vi "H2O_DIAL_NCAR_4CH_v4.07.vi"() -> ()   [LabVIEW 2012]
uses:
  C:/Users/H2ODial/Desktop/Shared Telescope WV DIAL Code/Libraries and VIs/PowerMeterCommands.dll
  Libraries and VIs/PowerMeterCommands.dll
  <vilib>/DAQmx/write.llb/DAQmx Write (Digital 1D Bool NChan 1Samp 1Line).vi
  <vilib>/DAQmx/miscellaneous.llb/DAQmx Fill In Error Info.vi
  <vilib>/Analysis/baseanly.llb/Mean (DBL).vi
  AMCS_Data.vi
  Libraries and VIs/Scalar_Data.vi
  <vilib>/Analysis/NI_AALBase.lvlib
  Libraries and VIs/Scalar_Data_2.vi
  Libraries and VIs/Scalar_Data_4.vi
  Libraries and VIs/Scalar_Data_3.vi
  Libraries and VIs/CLDevIFace.dll
panel:
  in  "Cancel Offline":bool
  out "AMCS_Profile":i32=9505
  out "FileHour":i32=21
  out "L_Count":i32=24
  out "sigma_off_total":dbl[](array[numeric])=[5.235525125067343e-25, 5.206358319245337e-25, 5.177318750524933e-25, 5.148406424862825e-25, 5.119621341127451e-25, 5.090963491196627e-25, 5.062432860011865e-25, 5.034029425635027e-25, 5.005753159352157e-25, 4.977604025706667e-25, 4.949581982592347e-25, 4.921686981325722e-25, 4.893918966711095e-25, 4.866277877122191e-25, 4.8387636445644285e-25, 4.811376194764721e-25, 4.784115447230487e-25, 4.756981315339233e-25, 4.729973706394386e-25, 4.703092521721628e-25, 4.6763376567211625e-25, 4.6497090009594435e-25, 4.623206438225019e-25, 4.596829846622293e-25, 4.57057909862005e-25, 4.544454061150213e-25, 4.518454595652437e-25, 4.492580558158126e-25, 4.4668317993693425e-25, 4.441208164702635e-25, 4.41570949437918e-25, 4.390335623482575e-25, 4.365086382028137e-25, 4.339961595028071e-25, 4.314961082547237e-25, 4.290084659777996e-25, 4.2653321370993085e-25, 4.240703320135042e-25, 4.216198009811418e-25, 4.191816002426457e-25, 4.16755708969195e-25, 4.143421058805604e-25, 4.1194076924960845e-25, 4.095516769084665e-25, 4.0717480625238245e-25, 4.0481013424706545e-25, 4.0245763743206737e-25, 4.001172919260011e-25, 3.977890734322512e-25, 3.9547295724256756e-25, 3.931689182419048e-25, 3.908769309139365e-25, 3.8859696934393876e-25, 3.863290072236815e-25, 3.840730178557474e-25, 3.8182897415734565e-25, 3.7959684866403156e-25, 3.773766135338825e-25, 3.7516824055099053e-25, 3.729717011286995e-25, 3.707869663137923e-25, 3.686140067893342e-25, 3.664527928779591e-25, 3.643032945453827e-25, 3.621654814033011e-25, 3.600393227122229e-25, 3.579247873843723e-25, 3.5582184398664743e-25, 3.5373046074361216e-25, 3.5165060553938904e-25, 3.4958224592064764e-25, 3.475253490990589e-25, 3.454798819536632e-25, 3.4344581103303625e-25, 3.414231025576395e-25, 3.394117224218377e-25, 3.37411636196096e-25, 3.3542280912885406e-25, 3.3344520614845767e-25, 3.3147879186525413e-25, 3.295235305730259e-25, 3.275793862509532e-25, 3.2564632256504646e-25, 3.237243028702917e-25, 3.2181329021119735e-25, 3.1991324732434905e-25, 3.180241366390581e-25, 3.161459202790299e-25, 3.142785600633377e-25, 3.1242201750825597e-25, 3.1057625382770893e-25, 3.0874122993477767e-25, 3.0691690644282785e-25, 3.051032436660927e-25, 3.0330020162078266e-25, 3.0150774002602592e-25, 2.997258183045521e-25, 2.979543955833093e-25, 2.961934306943937e-25, 2.944428821752431e-25, 2.9270270826932477e-25, 2.909728669267514e-25, 2.8925331580414936e-25, 2.875440122654977e-25, 2.8584491338173137e-25, 2.841559759313169e-25, 2.8247715639976386e-25, 2.80808410980223e-25, 2.791496955724979e-25, 2.775009657833479e-25, 2.7586217692567447e-25, 2.742332840183121e-25, 2.7261424178518227e-25, 2.710050046547509e-25, 2.6940552675881075e-25, 2.6781576193155516e-25, 2.6623566370876434e-25, 2.646651853260364e-25, 2.6310427971768174e-25, 2.615528995144771e-25, 2.600109970428841e-25, 2.5847852432207883e-25, 2.569554330624564e-25, 2.554416746633416e-25, 2.5393720020962457e-25, 2.5244196047033826e-25, 2.5095590589459477e-25, 2.4947898660936654e-25, 2.480111524155541e-25, 2.4655235278440513e-25, 2.451025368544176e-25, 2.436616534266772e-25, 2.422296509605852e-25, 2.408064775697375e-25, 2.3939208101763006e-25, 2.3798640871112015e-25, 2.365894076971971e-25, 2.352010246556833e-25, 2.3382120589521406e-25, 2.324498973455175e-25, 2.3108704455300754e-25, 2.2973259267270024e-25, 2.283864864626908e-25, 2.270486702764721e-25, 2.257190880557015e-25, 2.2439768332388837e-25, 2.2308439917739663e-25, 2.2177917827749597e-25, 2.20481962844103e-25, 2.19192694645104e-25, 2.179113149897461e-25, 2.166377647190967e-25, 2.153719841983278e-25, 2.1411391330535246e-25, 2.1286349142540036e-25, 2.1162065743868337e-25, 2.103853497130775e-25, 2.091575060946101e-25, 2.079370638983031e-25, 2.0672395989815037e-25, 2.0551813031976677e-25, 2.0431951082869756e-25, 2.0312803652523447e-25, 2.019436419319984e-25, 2.0076626098781596e-25, 1.9959582703908636e-25, 1.9843227283026113e-25, 1.9727553050009988e-25, 1.9612553156963306e-25, 1.9498220693936616e-25, 1.9384548688025462e-25, 1.9271530103114487e-25, 1.915915783921294e-25, 1.9047424731896738e-25, 1.8936323552292957e-25, 1.8825847006561212e-25, 1.8715987735714719e-25, 1.8606738315918164e-25, 1.8498091257941087e-25, 1.8390039007904753e-25, 1.8282573946936752e-25, 1.8175688392200846e-25, 1.80693745969556e-25, 1.7963624751388698e-25, 1.7858430983630522e-25, 1.7753785360393623e-25, 1.7649679888396773e-25, 1.7546106515613228e-25, 1.7443057132789558e-25, 1.7340523575155863e-25, 1.723849762422857e-25, 1.7136971010131167e-25, 1.7035935413825008e-25, 1.6935382469544605e-25, 1.6835303767796407e-25, 1.6735690858143057e-25, 1.6636535252563445e-25, 1.653782842907513e-25, 1.643956183497921e-25, 1.6341726891478545e-25, 1.624431499756322e-25, 1.6147317534796005e-25, 1.6050725871551994e-25, 1.5954531368896971e-25, 1.585872538492723e-25, 1.576329928151117e-25, 1.566824442883223e-25, 1.5573552212546758e-25, 1.5479214039898043e-25, 1.5385221346219397e-25, 1.5291565602013113e-25, 1.519823831962039e-25, 1.5105231061650234e-25, 1.5012535447460145e-25, 1.49201431624485e-25, 1.482804596459418e-25, 1.4736235693849326e-25, 1.46447042805166e-25, 1.455344375360034e-25, 1.4462446250285657e-25, 1.4371704024629248e-25, 1.4281209456557682e-25, 1.4190955061389853e-25, 1.410093350012645e-25, 1.4011137586880333e-25, 1.3921560301221658e-25, 1.3832194795253431e-25, 1.3743034404767374e-25, 1.3654072658699072e-25, 1.3565303288298996e-25, 1.3476720236918642e-25, 1.3388317669734332e-25, 1.3300089982893968e-25, 1.3212031812258562e-25, 1.3124138043688156e-25, 1.3036403820696332e-25, 1.2948824553577423e-25, 1.2861395928315612e-25, 1.2774113913410786e-25, 1.2686974768684636e-25, 1.2599975053009544e-25, 1.2513111630057894e-25, 1.2426381676023619e-25, 1.2339782685325752e-25, 1.2253312476934588e-25, 1.2166969199403071e-25, 1.2080751335374065e-25, 1.1994657705541538e-25, 1.1908687474046665e-25, 1.182284014933639e-25, 1.1737115587808914e-25, 1.1651513996305814e-25, 1.1566035931942852e-25, 1.1480682304187532e-25, 1.1395454373665928e-25, 1.1310353751750977e-25, 1.1225382399779688e-25, 1.1140542626706877e-25, 1.1055837085176348e-25, 1.097126877076807e-25, 1.0886841014622313e-25, 1.0802557481625692e-25, 1.07184221622742e-25, 1.0634439369229237e-25, 1.0550613727868173e-25, 1.0466950171251473e-25, 1.038345393031225e-25, 1.0300130526116006e-25, 1.0216985760646603e-25, 1.0134025706453978e-25, 1.0051256696943142e-25, 9.968685315566847e-26, 9.886318383691271e-26, 9.804162950309608e-26, 9.722226278487634e-26, 9.640515833439737e-26, 9.559039270504641e-26]
  out "sigma_on_total":dbl[](array[numeric])=[2.0626424870063408e-23, 2.0548386991725913e-23, 2.0469620043661083e-23, 2.039014007926666e-23, 2.0309963185763554e-23, 2.022910547933105e-23, 2.0147583096531975e-23, 2.0065412185834914e-23, 1.9982608903424648e-23, 1.9899189402652408e-23, 1.9815169828925073e-23, 1.973056631280819e-23, 1.9645394962489817e-23, 1.9559671857889236e-23, 1.9473413042995686e-23, 1.9386634520995392e-23, 1.9299352246499e-23, 1.92115821209391e-23, 1.9123339984701628e-23, 1.9034641613560593e-23, 1.894550271072393e-23, 1.8855938903179933e-23, 1.8765965734424238e-23, 1.8675598661476663e-23, 1.858485304716652e-23, 1.8493744158198464e-23, 1.8402287157379186e-23, 1.831049710049574e-23, 1.8218388932961533e-23, 1.8125977482532266e-23, 1.8033277457757753e-23, 1.794030344287124e-23, 1.78470698943209e-23, 1.7753591137085564e-23, 1.765988136004934e-23, 1.756595461410152e-23, 1.7471824808549346e-23, 1.737750570768982e-23, 1.728301092753991e-23, 1.718835393452682e-23, 1.7093548040708237e-23, 1.6998606403479167e-23, 1.690354202181418e-23, 1.6808367735172782e-23, 1.671309621933486e-23, 1.6617739987721353e-23, 1.652231138715337e-23, 1.6426822596607076e-23, 1.6331285627143943e-23, 1.623571231880846e-23, 1.614011433977554e-23, 1.6044503186999793e-23, 1.594889018281904e-23, 1.5853286475164595e-23, 1.5757703037183567e-23, 1.56621506662899e-23, 1.5566639983337563e-23, 1.5471181432924705e-23, 1.5375785282782344e-23, 1.5280461622943503e-23, 1.5185220367027678e-23, 1.5090071251272868e-23, 1.4995023834679822e-23, 1.490008749990639e-23, 1.480527145325558e-23, 1.4710584724761487e-23, 1.461603616869313e-23, 1.4521634464462555e-23, 1.4427388117922844e-23, 1.4333305460496324e-23, 1.4239394650957737e-23, 1.4145663676315014e-23, 1.4052120352758215e-23, 1.3958772326362732e-23, 1.386562707448506e-23, 1.377269190659265e-23, 1.3679973965774194e-23, 1.3587480229685293e-23, 1.349521751185974e-23, 1.340319246367332e-23, 1.331141157483609e-23, 1.3219881175450048e-23, 1.312860743690352e-23, 1.303759637488782e-23, 1.2946853848301087e-23, 1.2856385563810112e-23, 1.276619707542367e-23, 1.2676293787044932e-23, 1.2586680953306706e-23, 1.2497363683020601e-23, 1.2408346938918898e-23, 1.231963554057768e-23, 1.2231234166482255e-23, 1.2143147354716326e-23, 1.205537950536109e-23, 1.1967934882614928e-23, 1.18808176163727e-23, 1.179403170382724e-23, 1.1707581012163646e-23, 1.1621469279366376e-23, 1.1535700116662612e-23, 1.1450277010949764e-23, 1.1365203325379191e-23, 1.1280482302846387e-23, 1.119611706633001e-23, 1.1112110622106432e-23, 1.1028465860371398e-23, 1.0945185558937296e-23, 1.0862272383097774e-23, 1.0779728889052267e-23, 1.0697557524793115e-23, 1.061576063274372e-23, 1.0534340451140567e-23, 1.0453299116394038e-23, 1.0372638664219593e-23, 1.0292361031742144e-23, 1.0212468060051632e-23, 1.0132961495072904e-23, 1.0053842990094956e-23, 9.975114106406274e-24, 9.896776316950593e-24, 9.818831006241923e-24, 9.741279473284931e-24, 9.664122933306695e-24, 9.587362518136572e-24, 9.510999279944331e-24, 9.4350341911426e-24, 9.35946814739855e-24, 9.284301968408356e-24, 9.209536399550346e-24, 9.135172114369533e-24, 9.061209715316372e-24, 8.987649735342966e-24, 8.914492639894921e-24, 8.841738828863562e-24, 8.769388636455937e-24, 8.697442334770948e-24, 8.625900133437759e-24, 8.554762182711667e-24, 8.484028573306861e-24, 8.413699339425238e-24, 8.343774458768281e-24, 8.274253854911725e-24, 8.20513739808004e-24, 8.136424906498288e-24, 8.068116148476333e-24, 8.000210842753849e-24, 7.93270865979759e-24, 7.865609224179398e-24, 7.798912114328467e-24, 7.732616864864992e-24, 7.666722967246401e-24, 7.601229871485918e-24, 7.536136986062991e-24, 7.47144368084401e-24, 7.407149286604625e-24, 7.343253097014758e-24, 7.279754369538433e-24, 7.216652326491339e-24, 7.153946155744344e-24, 7.091635012419465e-24, 7.029718018888616e-24, 6.968194267085294e-24, 6.907062818145217e-24, 6.846322704177098e-24, 6.785972929020363e-24, 6.726012468678494e-24, 6.666440273317614e-24, 6.607255266717305e-24, 6.5484563482276464e-24, 6.490042392830114e-24, 6.4320122527255365e-24, 6.374364757672102e-24, 6.317098715478381e-24, 6.260212913519775e-24, 6.203706118893361e-24, 6.147577079162962e-24, 6.091824523799792e-24, 6.036447163734017e-24, 5.981443693189575e-24, 5.9268127892254286e-24, 5.872553113518711e-24, 5.818663312168178e-24, 5.765142016606135e-24, 5.711987844480541e-24, 5.659199399714517e-24, 5.60677527349843e-24, 5.554714044726636e-24, 5.503014280556554e-24, 5.451674536954151e-24, 5.400693359100156e-24, 5.3500692821650106e-24, 5.29980083168557e-24, 5.249886523936265e-24, 5.200324866659172e-24, 5.151114359286823e-24, 5.102253493524346e-24, 5.053740753912813e-24, 5.0055746177903024e-24, 4.9577535563097775e-24, 4.9102760344956494e-24, 4.8631405118766655e-24, 4.816345442421003e-24, 4.769889275599373e-24, 4.7237704559666584e-24, 4.677987424414909e-24, 4.6325386175288775e-24, 4.587422468700435e-24, 4.542637408235811e-24, 4.498181863571078e-24, 4.454054259692367e-24, 4.410253019129813e-24, 4.366776562876656e-24, 4.323623309953703e-24, 4.2807916785034235e-24, 4.238280085149713e-24, 4.196086945869007e-24, 4.15421067614052e-24, 4.112649690999126e-24, 4.0714024055659475e-24, 4.030467235085202e-24, 3.989842595058185e-24, 3.949526901559562e-24, 3.9095185718135265e-24, 3.8698160234810635e-24, 3.830417676044675e-24, 3.7913219499109044e-24, 3.752527267230076e-24, 3.7140320519806624e-24, 3.675834729967747e-24, 3.6379337290799074e-24, 3.600327479534733e-24, 3.563014413948001e-24, 3.525992967320637e-24, 3.489261577597712e-24, 3.4528186853946936e-24, 3.416662734299426e-24, 3.380792171158687e-24, 3.345205445806531e-24, 3.309901011503899e-24, 3.2748773251256216e-24, 3.240132846887192e-24, 3.205666040760562e-24, 3.171475374424784e-24, 3.1375593195130495e-24, 3.103916351630131e-24, 3.070544950370658e-24, 3.0374435993380817e-24, 3.004610786651537e-24, 2.9720450044576056e-24, 2.939744749292133e-24, 2.907708522285371e-24, 2.875934828888819e-24, 2.8444221792793013e-24, 2.813169088151738e-24, 2.7821740748481583e-24, 2.751435663542785e-24, 2.7209523832266658e-24, 2.6907227675070794e-24, 2.6607453552206828e-24, 2.631018689789545e-24, 2.601541319883231e-24, 2.5723117989072515e-24, 2.5433286855837636e-24, 2.514590543447409e-24, 2.4860959413513324e-24, 2.4578434531440932e-24, 2.4298316578731105e-24, 2.402059139807656e-24, 2.3745244883501128e-24, 2.3472262981695396e-24, 2.3201631692184444e-24, 2.2933337065889e-24, 2.2667365207963308e-24, 2.240370227526033e-24, 2.2142334477539052e-24, 2.188324807908419e-24]
  out "background start":u32=269
  in  "Tab Control 2":enum32{"WV ND far", "WV ND near"}(tab)
  out "Water Vapor Number Density":dbl[][](graph)=[[1.0639074632249623, 0.7950854451951521, 0.6871802900906222, 0.6578628096137078, 0.7135791866585837, 0.791964119748022, 0.7860957670990096, 0.7853422876996722, 0.8071252522931472, 0.8864535505893456, 1.0159198981230433, 0.9651627659284989, 0.8682042083486436, 0.9042154310622283, 0.8685330628018557, 0.7776092079248705, 0.772778664796884, 0.7959779985601635, 0.8008645625247376, 0.7172845453518656, 0.6359963863515634, 0.7577960001972899, 0.7813956634686308, 0.6712364496556374, 0.799991558752808, 0.8995446623945136, 0.8463956496056573, 0.9017639404246155, 0.6968132420137522, 0.4583190307261309, 0.9013318132552974, 0.9419840408259437, 0.2861834314217356, 0.4216587338337765, 0.874217351771625, 0.8730810394400317, 1.1849849949997056, 0.877588935205842, -0.09895312689728929, 0.2099354782570955, 0.33582425948864986, 0.3612751226151659, 0.28889957151168794, 0.27667685078031906, -0.08105679033755347, -0.25446230513135015, -0.2766196124323003, -0.18163086301089895, 0.12220991421169942, 0.48573696212417655, 0.648089394728748, 0.7347271367978115, 0.548882739398166, 0.33491079910936744, 0.6580156316208491, 0.8064375648282445, 0.8640275078789249, 0.8753236062578905, 0.6701265812361802, 0.3904351761194603, 0.24849863279105913, 0.09000958662382388, 0.265877091881824, 0.5782261463654136, 0.6582345385490979, 0.5377226976111342, 0.521998023122092, 0.49899994069903986, 0.442086244580199, 0.7757271869672275, 1.6438430791775833, 1.7725263534215783, -4.366638673239888, -6.139974535528756, -7.260343261365436, -3.647297503921928, 2.5607177071489544, -3.1758534783949344, -4.1712374154778065, -4.871973805244922, -7.278334464601457, -6.425192249591581, -2.0047084004412903, 2.3698571856595816, 7.6963844059742055, 2.29139948545028, -6.73627824143711, -2.991965195732426, 3.0525104440963333, 3.2900333489586076, -1.1469438869155248, -2.480793373210193, 2.985721257146301, 6.404469953330058, 2.223833509425413, -3.3828689101014184, -0.7090064353515616, 1.7614922219798188, -10.376535524618875, -5.53316518310933, -1.3807982250792938, -4.60098490166722, 7.202468070896515, 26.808797183465867, -5.359274301526265, 5.1064602266204036, 8.904280843443795, 5.443742898428987, 12.764870740289377, 5.608742098911494, 9.23856034631878, 13.494920524668304, -1.6256568257766502, -27.752190916852243, 4.922130515696406, 1.2918095411038983, -2.2167544171775706, 3.8512090071660414, 0.8411143725920815, 2.3628258559477175, -0.0338690724559584, 0.5037405048509485, 0.857274736311794, 0.5609093472806994, 0.38332080391643575, 1.2134171316753553, 5.4760246071133345, 10.097061664150369, 14.664568150924406, -9.066581270887879, 3.8358908500396702, -4.8511138822779785, -2.9839925207514213, 10.022780631409056, 1.4845952961432987, 1.3621427534838009, -11.797751493789379, -19.62876466384785, -15.407318505260495, 12.982964456880289, -28.114070918045577, -10.314928052994132, -14.6863478886457, -7.4678357637899575, 8.005743163091363, -4.049991074487799, 3.834478174499156, 1.9703319457006785, -18.69907677622087, -21.61726008053773, 17.044786369322896, 13.067986458307882, 5.562083807824563, -33.1062622690423, -18.99604811314825, -14.780095581334582, -9.038972930950822, 25.682641251556422, 29.060493890117453, 30.197267081841407, 0.1585102430855488, -19.120769948554525, -50.066668611302525, 6.80906230633824, -36.08725775608675, -13.983058385627226, -11.304401633639582, -45.42704769175601, 4.201427809981585, -29.24086259807242, 18.154194101391802, 22.333042820598845, 45.23184778962592, 8.205432492461684, 36.41380298442893, 31.12103406953646, 8.501419515989362, 4.038593181058191, -39.965946639630644, 23.376757826064956, -12.263734474568551, -9.673975161682188, -1.2694403063797983, 31.516249824703433, 26.931341924650482, -12.240477775714073, -9.145842740233656, 4.271762269200702, 28.58651015280052, 22.54270081951647, -10.57215914472278, -0.9151487571192986, 1.767320075481733, -8.699514625176734, -36.202725126831716, 7.3259828957797914, 20.584536573322936, 4.297763618632405, -7.114175066775342, -41.052676712996984, 4.575962205650572, -16.179022663355003, -4.304361509159662, -22.29272241704299, 5.168440976430942, -4.301060404937512, 5.910531683494024, 13.869916287008905, 3.299425512420319, -10.2596400971753, -15.98556021271673, -21.119499530599604, 10.121801879771763, 17.07162378753489, 21.60248052204745, -44.7136046984398, -69.32086239761064, -8.665106806341068, 10.787462206990869, 30.84192690886579, -62.81604147152294, 68.55391085081732, 8.457719191474123, -28.577047707128873, 38.603673426774556, 61.94525626705892, 33.58700658348496, -1.9078968009888306, -32.30145114234005, -18.09981763911342, 88.5341483784121, -53.75429796396262, -12.113128819524603, -20.864631528502642, -53.546127210198485, 19.394365608128517, 26.53767479667509, -6.401595356851402, -61.36866888555028, -67.51786171355864, 2.78000703125268, 76.33614125496274, -35.64199728183781, 4.150760130500163, -4.696052234502958, -64.62075727916867, -9.689952747671516, 30.355740029469093, 158.13941477463777, 84.62554961101615, 37.37518451892517, -19.315848810070918, 22.407516333304084, 38.17938221937312, 19.600756478441497, 45.386701820912904, 51.438745402980494, 8.749021339340636, -91.86439146049418, 9.144403904105646, -34.267323390646695, -74.3567957578877, 39.32846577092227, 50.75034914631157, -10.066496831755677, 85.8002054961762, -10.499894043979156, 14.390636790059602, 68.28171532154174, 22.15122916807249, 14.907521727984179, 71.39835561945517, 9.422251399802613, -23.7765608484535, 23.347606952235623, -72.28850134204748, 0.0, 0.0, 0.0, 0.0]]
  out "Water Vapor Number Density 2":dbl[][](graph)=[[nan, nan, nan, nan, nan, nan, nan, nan, nan, nan, nan, nan, nan, nan, nan, nan, nan, nan, nan, nan, nan, nan, nan, nan, nan, nan, nan, nan, nan, nan, nan, nan, nan, nan, nan, nan, nan, nan, nan, nan, nan, nan, nan, nan, nan, nan, nan, nan, nan, nan, nan, nan, nan, nan, nan, nan, nan, nan, nan, nan, nan, nan, nan, nan, nan, nan, nan, nan, nan, nan, nan, nan, nan, nan, nan, nan, nan, nan, nan, nan, nan, nan, nan, nan, nan, nan, nan, nan, nan, nan, nan, nan, nan, nan, nan, nan, nan, nan, nan, nan, nan, nan, nan, nan, nan, nan, nan, nan, nan, nan, nan, nan, nan, nan, nan, nan, nan, nan, nan, nan, nan, nan, nan, nan, nan, nan, nan, nan, nan, nan, nan, nan, nan, nan, nan, nan, nan, nan, nan, nan, nan, nan, nan, nan, nan, nan, nan, nan, nan, nan, nan, nan, nan, nan, nan, nan, nan, nan, nan, nan, nan, nan, nan, nan, nan, nan, nan, nan, nan, nan, nan, nan, nan, nan, nan, nan, nan, nan, nan, nan, nan, nan, nan, nan, nan, nan, nan, nan, nan, nan, nan, nan, nan, nan, nan, nan, nan, nan, nan, nan, nan, nan, nan, nan, nan, nan, nan, nan, nan, nan, nan, nan, nan, nan, nan, nan, nan, nan, nan, nan, nan, nan, nan, nan, nan, nan, nan, nan, nan, nan, nan, nan, nan, nan, nan, nan, nan, nan, nan, nan, nan, nan, nan, nan, nan, nan, nan, nan, nan, nan, nan, nan, nan, nan, nan, nan, nan, nan, nan, nan, nan, nan, nan, nan, nan, nan, nan, nan, nan, nan, nan, nan, nan, nan, nan, nan, 0.0, 0.0, 0.0, 0.0]] caption="Water Vapor Number Density"
  out "RingBuffer offline near":dbl[][](array[numeric])
  out "RingBuffer aerosol near":dbl[][](array[numeric])
  in  "?":T1(tab)=enum."Raw Counts far"
  out "NRB":dbl[][](graph)=[[0.00021949387338662354, 0.0012644243666972022, 0.003588214032197759, 0.007224875605591026, 0.01195486448906066, 0.017431459045268816, 0.02324525277374715, 0.028802949441434758, 0.03357339059910846, 0.03782380503740098, 0.04151485605543974, 0.04515843930280387, 0.049063338651475254, 0.05265022207418093, 0.05575153288521212, 0.058504265927874735, 0.06054542510466426, 0.06174893486130328, 0.06273751305790501, 0.0632643954466035, 0.06351151944448351, 0.06357989044996755, 0.06341560380273549, 0.06303851009419217, 0.062470398076431455, 0.06280916033724494, 0.06322756790340872, 0.06364161839774003, 0.06419606813751108, 0.06488643226694854, 0.06547481871569719, 0.06547690406532276, 0.0653459113875375, 0.06474035391034692, 0.06486724045628954, 0.06495721309884349, 0.06533471884747548, 0.06616972815999793, 0.06638610910810476, 0.06655916600871534, 0.06537078233011287, 0.06602313200264284, 0.07317302762243715, 0.09749970595442206, 0.16406250986720886, 0.2791180302249938, 0.4176438777801052, 0.6802666334717046, 1.1591238150403569, 1.8560464374847874, 3.875101405163791, 6.174829462839288, 7.153508037509122, 6.549121280175305, 4.477651124476559, 2.2218355272416597, 0.7640138940197323, 0.38355427091296046, 0.22127538753969628, 0.15301899733856175, 0.11710012281226226, 0.08146079585564299, 0.055184033492043434, 0.037862430693885785, 0.034092862578169306, 0.05242220252049839, 0.07432678147202534, 0.07994648052250543, 0.07740338358404796, 0.09601527433306305, 0.13781740302265783, 0.16817436004198102, 0.17204903952050793, 0.14666788769173048, 0.08534420683870735, 0.026147036283789102, 0.004856085115782482, 0.0011524972448401112, -0.0013581678605637906, -0.0003334964710556502, -0.00010807353538194676, -0.003124612121326412, -0.004336002492278915, -0.0014014221205421228, 0.0027475954822278555, 0.003000058320868829, -0.000784026500043395, -0.0036292638303861017, -0.0018994070353000377, -0.0022502258539117076, -0.0033235236994120262, -0.0002667745861222975, 0.002857604546389024, 0.0024085602442003792, 0.0008948278806142738, -0.004348316485827131, -0.0036123162720960353, -0.001093692801835954, -7.606460251392899e-05, 0.0001995662750162021, -0.0032458877310182544, -0.0067049146072067555, -0.011255959074133778, -0.0075100285269975465, -1.5715830895250584e-05, 0.0014521797234306707, 0.0017698492925668126, -0.0021134242858882064, -0.006198461561210931, 0.002272948224295056, 0.01583894655602962, 0.03911679247954582, 0.05065155756276627, 0.03434974415408211, 0.016131693983398827, 0.0015259742615324821, -0.0029356412127107072, 0.006441985833132487, 0.0067535033006338955, -0.002232846099778923, 0.0030169480576232905, 0.006072797187070327, 0.00840132753763888, 0.025648255839425066, 0.07154886818880388, 0.13144237654754948, 0.14147442902347296, 0.10060890346164576, 0.06881876829844959, 0.04548498306360664, 0.018363981113472608, 0.007178133641252553, 0.0006471905285573144, 0.00013082291360446007, -0.0003868015765336126, -0.0008319776309399116, -0.0032372953366313776, 0.003079661264735281, 0.0007528035169903232, -0.006857440598945683, -0.011190829128121376, -0.020132237433723756, -0.012449768687672693, -0.004430467301130137, -0.0045588153304884195, -0.007187731694288056, -0.008552841137992364, -0.0057034422030721, -0.0038995755277612646, 0.0026406996122382968, 0.0019898633505103873, -0.012364667965739512, -0.004352753118895328, -0.0026819703918430173, -0.005247351813261463, 0.008252545743437438, -0.00042554135370181706, -0.013261247816825816, -0.01437057771837057, -0.017613037229624345, -0.015329648358374798, -0.013109901231006636, -0.024991290073243147, -0.01028335129982454, -0.005170113537865864, -0.011255810708455646, -0.004015231795578576, -0.005471582128283474, 0.0004116530263236128, 0.002979866875647862, 0.0142463354607509, 0.015327191442677624, 0.005148032069807082, 0.008324711549857047, -0.0007954919041935178, -0.0104941333208857, -0.0038654329070212587, -0.0065438045583597225, -0.0146355737553841, -0.005870623016356129, -0.010346492671299242, -0.01279570499844253, 0.002657403663372611, -0.003185200259090592, -0.002189979195384867, 0.0029918256232875457, -0.0005483203986729846, 0.0005374071696337536, -0.018466354202582292, -0.03392773745655944, -0.020303701319439753, -0.014882696897406955, -0.006601732618584244, -0.007475045766542423, -0.013725356228314145, -0.0030666031317952477, 0.007536028196976982, -0.0018876410045178442, -0.013447494563607994, 0.008337497509276084, -0.0013373777621936394, -0.029592197421304763, -0.01056697775939752, 0.0018521820948973538, 0.0037341208592153487, 0.0007124540469122575, -0.012785942256115651, -0.00506390285966855, 0.005057410403679166, -0.020597837150005866, -0.041524722796550874, -0.005153764699711019, 0.012402834478974131, -0.010763999846621129, -0.019650264880285036, -0.009746865677268082, -0.013379913325527208, -0.02005193275862931, -0.017425758044107502, -0.01839015378175284, -0.014960704010900442, -0.002568131262422916, -0.01101894224132209, -0.017396108976988567, 0.01716737049069364, 0.026947396830469546, 0.002415797307856873, 0.008324149245365493, 0.015748192283591606, -0.0008294818007321022, 0.0008958728531738392, 0.01927520182779269, 0.010713947919074691, 0.00963529584292991, 0.029748690501360413, -0.0018877890483105903, -0.024322266576488477, -0.011878307635102106, -0.005419225989488603, -0.014952480732913196, -0.013697490395655548, -0.0011965651669468304, -0.01925659817402323, 0.010806464854841815, 0.018215837313548467, -0.009143916741043851, 0.036681465606137, 0.06201597020329838, 0.057999524678215446, 0.035350521579985146, -0.002285065048543413, 0.0018708147901757444, -0.0030312913687593613, -0.01424435165120654, -0.002152495952739822, -0.0031555055829017783, -0.018558005972215068, -0.03166995520900352, -0.0036017583361618926, 0.002633896679703226, -0.034460654338889354, -0.042226737046900734, 0.0009969408696396463, 0.05559343523719784, 0.028207470700457017, -0.009850675799292778, 0.004076120070937046, -0.011080061340762158, -0.030187659584441594, -0.02920019529217202, 0.00024427228639596057, -0.004734066348907353, -0.015215666336210342, 0.01921600632874382, 0.039839412543775904, 0.007975128364511024, -0.027088179548068966, 0.0, 0.0, 0.0]] caption="Water Vapor Number Density"
  out "NRB 2":dbl[][](graph) caption="Water Vapor Number Density"
  out "raw counts":dbl[][](graph)=[[886.0, 1449.0, 1867.0, 2250.0, 2322.0, 2310.0, 2337.0, 2109.0, 2024.0, 1831.0, 1806.0, 1607.0, 1504.0, 1357.0, 1172.0, 1199.0, 937.0, 1054.0, 864.0, 876.0, 727.0, 718.0, 698.0, 659.0, 591.0, 484.0, 481.0, 436.0, 479.0, 394.0, 412.0, 428.0, 375.0, 308.0, 324.0, 327.0, 267.0, 254.0, 296.0, 286.0, 225.0, 221.0, 193.0, 196.0, 227.0, 210.0, 204.0, 175.0, 410.0, 562.0, 3722.0, 28458.0, 28603.0, 11926.0, 302.0, 36.0, 53.0, -3.0, -1.0, 34.0, 2.0, 47.0, 38.0, -31.0, -51.0, 24.0, -28.0, 25.0, 72.0, -15.0, 6.0, 53.0, 7.0, 6.0, 46.0, 18.0, 28.0, 4.0, 30.0, 11.0, 51.0, 25.0, 0.0, -9.0, 33.0, 25.0, 28.0, 3.0, -15.0, 18.0, 13.0, -13.0, -20.0, 37.0, 27.0, -8.0, -53.0, -6.0, 20.0, -33.0, 14.0, -37.0, -62.0, 4.0, -2.0, 5.0, 27.0, 26.0, -28.0, -17.0, -51.0, -18.0, 17.0, 18.0, 15.0, -10.0, 10.0, 5.0, 39.0, 8.0, -21.0, -6.0, 59.0, -8.0, -24.0, 14.0, -3.0, 17.0, -14.0, -16.0, -10.0, 82.0, 16.0, -23.0, 53.0, 16.0, 13.0, -35.0, 40.0, 19.0, 14.0, 27.0, 45.0, 28.0, 6.0, 40.0, 22.0, -12.0, 46.0, 20.0, 17.0, -28.0, 4.0, 16.0, 8.0, -4.0, 61.0, 8.0, -17.0, -13.0, -58.0, 8.0, -14.0, -53.0, 28.0, 4.0, 2.0, -20.0, -12.0, 32.0, 19.0, 33.0, -34.0, 7.0, -23.0, 20.0, -23.0, 19.0, 24.0, -18.0, 10.0, 81.0, 19.0, -10.0, 18.0, -19.0, 54.0, 82.0, 23.0, 38.0, 11.0, -15.0, -20.0, 58.0, 34.0, 2.0, -22.0, 24.0, 25.0, 34.0, 21.0, -27.0, -22.0, -2.0, 12.0, -21.0, 42.0, -9.0, -42.0, 7.0, -33.0, 23.0, -6.0, -23.0, -38.0, 8.0, 9.0, -20.0, -25.0, 11.0, 30.0, -13.0, 27.0, 5.0, 2.0, 34.0, 6.0, 69.0, 18.0, -15.0, -17.0, -5.0, 54.0, -24.0, 45.0, -31.0, 0.0, 3.0, 53.0, 15.0, 61.0, 24.0, -32.0, 10.0, 31.0, -37.0, -20.0, 45.0, 65.0, 17.0, 12.0, -6.0, 44.0, -4.0, -4.0, 1.0, 29.0, 34.0, 17.0, 51.0, 0.0, 1.0, 38.0, 50.0, -48.0, -4.0, 6.0, 36.0, 29.0, -37.0, 44.0, -14.0, -36.0, -12.0, -4.0, 26.0, 10.0, -29.0, 52.0, 0.0]] caption="Water Vapor Number Density"
  out "raw counts near":dbl[][](graph) caption="Water Vapor Number Density"
  out "Aerosol Smoothed 2":dbl[](array[numeric])
  out "Off-Line Smoothed 2":dbl[](array[numeric])
  out "Off-Line Bin Readings 2":dbl[](array[numeric])
  out "On-Line Smoothed 2":dbl[](array[numeric])
  out "On-Line Bin Readings 2":dbl[](array[numeric])
  in  "stop":bool
  in  "Reset Average":bool=TRUE
  in  "Save Data?":bool=TRUE
  in  "Collect Data?":bool=TRUE
  in  "ILX Address":i32=6 min=0 step=1
  in  "Lambda On DBR Current":dbl=169.77999999999992
  in  "Lambda Off DBR Current":dbl=172.5300000000001
  in  "Tab Control":T2(tab)=enum."g/m^3"
  out "Water Vapor Number Density  2":cluster{"Y":dbl[], "Y":dbl[]}[](graph)=[{"Y"=array[276 elements], "Y"=array[280 elements]}, {"Y"=[nan, nan, nan, nan, nan, nan, nan, nan, nan, nan, nan, nan, nan, nan, nan, nan, nan, nan, nan, nan, nan, nan, nan, nan, nan, nan, nan, nan, nan, nan, nan, nan, nan, nan, nan, nan, nan, nan, nan, nan, nan, nan, nan, nan, nan, nan, nan, nan, nan, nan, nan, nan, nan, nan, nan, nan, nan, nan, nan, nan, nan, nan, nan, nan, nan, nan, nan, nan, nan, nan, nan, nan, nan, nan, nan, nan, nan, nan, nan, nan, nan, nan, nan, nan, nan, nan, nan, nan, nan, nan, nan, nan, nan, nan, nan, nan, nan, nan, nan, nan, nan, nan, nan, nan, nan, nan, nan, nan, nan, nan, nan, nan, nan, nan, nan, nan, nan, nan, nan, nan, nan, nan, nan, nan, nan, nan, nan, nan, nan, nan, nan, nan, nan, nan, nan, nan, nan, nan, nan, nan, nan, nan, nan, nan, nan, nan, nan, nan, nan, nan, nan, nan, nan, nan, nan, nan, nan, nan, nan, nan, nan, nan, nan, nan, nan, nan, nan, nan, nan, nan, nan, nan, nan, nan, nan, nan, nan, nan, nan, nan, nan, nan, nan, nan, nan, nan, nan, nan, nan, nan, nan, nan, nan, nan, nan, nan, nan, nan, nan, nan, nan, nan, nan, nan, nan, nan, nan, nan, nan, nan, nan, nan, nan, nan, nan, nan, nan, nan, nan, nan, nan, nan, nan, nan, nan, nan, nan, nan, nan, nan, nan, nan, nan, nan, nan, nan, nan, nan, nan, nan, nan, nan, nan, nan, nan, nan, nan, nan, nan, nan, nan, nan, nan, nan, nan, nan, nan, nan, nan, nan, nan, nan, nan, nan, nan, nan, nan, nan, nan, nan, nan, nan, nan, nan, nan, nan], "Y"=array[280 elements]}]
  out "Absolute Humidity":cluster{"Y":dbl[], "Y":dbl[]}[](graph)=[{"Y"=array[276 elements], "Y"=array[280 elements]}, {"Y"=[nan, nan, nan, nan, nan, nan, nan, nan, nan, nan, nan, nan, nan, nan, nan, nan, nan, nan, nan, nan, nan, nan, nan, nan, nan, nan, nan, nan, nan, nan, nan, nan, nan, nan, nan, nan, nan, nan, nan, nan, nan, nan, nan, nan, nan, nan, nan, nan, nan, nan, nan, nan, nan, nan, nan, nan, nan, nan, nan, nan, nan, nan, nan, nan, nan, nan, nan, nan, nan, nan, nan, nan, nan, nan, nan, nan, nan, nan, nan, nan, nan, nan, nan, nan, nan, nan, nan, nan, nan, nan, nan, nan, nan, nan, nan, nan, nan, nan, nan, nan, nan, nan, nan, nan, nan, nan, nan, nan, nan, nan, nan, nan, nan, nan, nan, nan, nan, nan, nan, nan, nan, nan, nan, nan, nan, nan, nan, nan, nan, nan, nan, nan, nan, nan, nan, nan, nan, nan, nan, nan, nan, nan, nan, nan, nan, nan, nan, nan, nan, nan, nan, nan, nan, nan, nan, nan, nan, nan, nan, nan, nan, nan, nan, nan, nan, nan, nan, nan, nan, nan, nan, nan, nan, nan, nan, nan, nan, nan, nan, nan, nan, nan, nan, nan, nan, nan, nan, nan, nan, nan, nan, nan, nan, nan, nan, nan, nan, nan, nan, nan, nan, nan, nan, nan, nan, nan, nan, nan, nan, nan, nan, nan, nan, nan, nan, nan, nan, nan, nan, nan, nan, nan, nan, nan, nan, nan, nan, nan, nan, nan, nan, nan, nan, nan, nan, nan, nan, nan, nan, nan, nan, nan, nan, nan, nan, nan, nan, nan, nan, nan, nan, nan, nan, nan, nan, nan, nan, nan, nan, nan, nan, nan, nan, nan, nan, nan, nan, nan, nan, nan, nan, nan, nan, nan, nan, nan], "Y"=array[280 elements]}]
  out "NRB plot":cluster{"Y":dbl[], "Y":dbl[]}[](graph)
  in  "background length":i32=10
  out "Correction":cluster{"Y":dbl[], "Y":dbl[]}[](graph)=[{"Y"=array[277 elements], "Y"=array[280 elements]}, {"Y"=[1.0, 1.0, 1.0, 1.0, 1.0, 1.0, 1.0, 1.0, 1.0, 1.0, 1.0, 1.0, 1.0, 1.0, 1.0, 1.0, 1.0, 1.0, 1.0, 1.0, 1.0, 1.0, 1.0, 1.0, 1.0, 1.0, 1.0, 1.0, 1.0, 1.0, 1.0, 1.0, 1.0, 1.0, 1.0, 1.0, 1.0, 1.0, 1.0, 1.0, 1.0, 1.0, 1.0, 1.0, 1.0, 1.0, 1.0, 1.0, 1.0, 1.0, 1.0, 1.0, 1.0, 1.0, 1.0, 1.0, 1.0, 1.0, 1.0, 1.0, 1.0, 1.0, 1.0, 1.0, 1.0, 1.0, 1.0, 1.0, 1.0, 1.0, 1.0, 1.0, 1.0, 1.0, 1.0, 1.0, 1.0, 1.0, 1.0, 1.0, 1.0, 1.0, 1.0, 1.0, 1.0, 1.0, 1.0, 1.0, 1.0, 1.0, 1.0, 1.0, 1.0, 1.0, 1.0, 1.0, 1.0, 1.0, 1.0, 1.0, 1.0, 1.0, 1.0, 1.0, 1.0, 1.0, 1.0, 1.0, 1.0, 1.0, 1.0, 1.0, 1.0, 1.0, 1.0, 1.0, 1.0, 1.0, 1.0, 1.0, 1.0, 1.0, 1.0, 1.0, 1.0, 1.0, 1.0, 1.0, 1.0, 1.0, 1.0, 1.0, 1.0, 1.0, 1.0, 1.0, 1.0, 1.0, 1.0, 1.0, 1.0, 1.0, 1.0, 1.0, 1.0, 1.0, 1.0, 1.0, 1.0, 1.0, 1.0, 1.0, 1.0, 1.0, 1.0, 1.0, 1.0, 1.0, 1.0, 1.0, 1.0, 1.0, 1.0, 1.0, 1.0, 1.0, 1.0, 1.0, 1.0, 1.0, 1.0, 1.0, 1.0, 1.0, 1.0, 1.0, 1.0, 1.0, 1.0, 1.0, 1.0, 1.0, 1.0, 1.0, 1.0, 1.0, 1.0, 1.0, 1.0, 1.0, 1.0, 1.0, 1.0, 1.0, 1.0, 1.0, 1.0, 1.0, 1.0, 1.0, 1.0, 1.0, 1.0, 1.0, 1.0, 1.0, 1.0, 1.0, 1.0, 1.0, 1.0, 1.0, 1.0, 1.0, 1.0, 1.0, 1.0, 1.0, 1.0, 1.0, 1.0, 1.0, 1.0, 1.0, 1.0, 1.0, 1.0, 1.0, 1.0, 1.0, 1.0, 1.0, 1.0, 1.0, 1.0, 1.0, 1.0, 1.0, 1.0, 1.0, 1.0, 1.0, 1.0, 1.0, 1.0, 1.0, 1.0, 1.0, 1.0, 1.0, 1.0, 1.0, 1.0, 1.0, 1.0, 1.0, 1.0, 1.0, 1.0, 1.0, 1.0, 1.0, 1.0, 1.0, 1.0, 1.0, 1.0, 1.0, 1.0, 1.0, 1.0, 1.0, 1.0, 1.0, 1.0, 1.0, 1.0], "Y"=array[280 elements]}]
  in  "dead time":dbl=3.7e-08
  out "Optical Depth":cluster{"Y":dbl[], "Y":dbl[]}[](graph) caption="XY Graph"
  out "RingBuffer offline far":dbl[][](array[numeric])
  out "RingBuffer aerosol far":dbl[][](array[numeric])
  in  "Weather":T3(tab)=enum."Pulse Energy (Micro Joule)"
  in  "Temperature (C)":dbl=15.0
  out "Temperature (C)":dbl(graph)=15.0
  in  "Pressure (mbar or hPa)":dbl=832.0
  out "Pressure (mb)":dbl(graph)=832.0
  out "Relative Humdity (%)":dbl(graph)=40.0
  out "Pulse Energy (Micro Joule)":T4(graph)={"Online Pulse Energy"=4.70368, "Pulse Energy Offline"=4.698567142857143}
  out "?":cluster{"mean":dbl, "mean":dbl}(graph)={"mean"=140400.0, "mean"=0.0}
  out "Index":i32=25
  out "Aerosol Smoothed":dbl[](array[numeric])=[1154.5512605042018, 1656.4756302521005, 2082.5344537815117, 2353.832773109242, 2490.1268907563012, 2520.849579831932, 2470.6941176470577, 2346.10588235294, 2163.7151260504193, 1977.2739495798314, 1796.0302521008398, 1643.5050420168066, 1522.857983193277, 1410.265546218487, 1301.9210084033612, 1201.6689075630252, 1102.412605042017, 1003.6142857142861, 915.7739495798323, 833.9378151260507, 759.7823529411769, 693.3705882352946, 633.0344537815129, 578.1605042016809, 528.2277310924371, 491.16050420168085, 458.59747899159674, 429.3117647058824, 403.7781512605043, 381.42941176470595, 360.51344537815135, 338.4000000000001, 317.61428571428576, 296.4798319327731, 280.36218487394956, 265.3999999999999, 252.73193277310912, 242.6857142857142, 231.1731092436974, 220.34957983193266, 206.0092436974789, 198.2865546218486, 209.6394957983192, 266.6689075630252, 428.4840336134455, 696.2319327731095, 995.6773109243697, 1548.467226890756, 2513.492436974789, 3826.8663865546205, 7465.6184873949605, 11114.20672268908, 12277.534453781518, 10945.820168067232, 7420.000840336137, 3656.752941176471, 1236.1647058823528, 602.223529411765, 336.4168067226891, 225.13949579831922, 166.76134453781503, 112.34117647058822, 73.72773109243698, 49.02605042016809, 42.799159663865574, 63.8201680672269, 87.790756302521, 91.66890756302521, 86.20252100840335, 103.88319327731091, 144.8957983193277, 171.89999999999992, 171.0764705882352, 141.95462184873944, 80.45042016806724, 24.013445378151275, 4.345378151260503, 1.005042016806721, -1.1546218487394977, -0.276470588235296, -0.0873949579831953, -2.465546218487397, -3.3394957983193296, -1.053781512605044, 2.017647058823527, 2.1521008403361326, -0.549579831932775, -2.4865546218487413, -1.2722689075630271, -1.4739495798319346, -2.129411764705884, -0.16722689075630448, 1.7529411764705864, 1.4462184873949562, 0.5260504201680652, -2.5033613445378173, -2.036974789915969, -0.6042016806722708, -0.04117647058823737, 0.10588235294117432, -1.688235294117649, -3.4193277310924386, -5.6294117647058854, -3.684033613445381, -0.007563025210085783, 0.6857142857142839, 0.820168067226889, -0.9613445378151283, -2.768067226890759, 0.9966386554621831, 6.820168067226888, 16.542857142857137, 21.04285714285714, 14.021848739495798, 6.471428571428569, 0.6016806722689056, -1.1378151260504223, 2.4546218487394937, 2.5302521008403343, -0.8226890756302541, 1.0932773109243676, 2.1647058823529393, 2.9462184873949564, 8.849579831932768, 24.29075630252102, 43.912605042016835, 46.52184873949583, 32.57226890756304, 21.93781512605041, 14.278151260504195, 5.6773109243697455, 2.185714285714284, 0.1941176470588217, 0.03865546218487212, -0.11260504201680865, -0.2386554621848759, -0.91512605042017, 0.8579831932773085, 0.20672268907562774, -1.8563025210084056, -2.9865546218487418, -5.297478991596641, -3.230252100840338, -1.1336134453781532, -1.1504201680672288, -1.7890756302521025, -2.1000000000000014, -1.3815126050420186, -0.9319327731092457, 0.6226890756302501, 0.46302521008403186, -2.8394957983193296, -0.9865546218487418, -0.6000000000000025, -1.1588235294117673, 1.7991596638655443, -0.09159663865546364, -2.8184873949579847, -3.0159663865546236, -3.650420168067228, -3.137815126050422, -2.650420168067229, -4.99075630252101, -2.0285714285714302, -1.007563025210086, -2.167226890756304, -0.7638655462184893, -1.0285714285714305, 0.07647058823529217, 0.5470588235294097, 2.58487394957983, 2.748739495798317, 0.9126050420168046, 1.4588235294117626, -0.13781512605042234, -1.797478991596641, -0.6546218487394979, -1.095798319327733, -2.423529411764708, -0.9613445378151281, -1.675630252100842, -2.0495798319327747, 0.4210084033613426, -0.49915966386554805, -0.3394957983193296, 0.45882352941176274, -0.08319327731092621, 0.08067226890756117, -2.7428571428571455, -4.986554621848742, -2.95294117647059, -2.1420168067226912, -0.9403361344537835, -1.0537815126050438, -1.91512605042017, -0.4235294117647078, 1.0302521008403343, -0.25546218487395167, -1.8016806722689096, 1.1058823529411748, -0.17563025210084215, -3.8478991596638674, -1.360504201680674, 0.2361344537815106, 0.4714285714285695, 0.08907563025209886, -1.5831932773109263, -0.6210084033613466, 0.6142857142857123, -2.4781512605042035, -4.948739495798321, -0.6084033613445397, 1.450420168067225, -1.2470588235294136, -2.2554621848739513, -1.10840336134454, -1.507563025210086, -2.2386554621848758, -1.9277310924369766, -2.0159663865546236, -1.6252100840336152, -0.27647058823529597, -1.1756302521008422, -1.8394957983193294, 1.7991596638655445, 2.7991596638655443, 0.24873949579831756, 0.8495798319327714, 1.593277310924368, -0.08319327731092618, 0.08907563025209903, 1.899999999999998, 1.0470588235294098, 0.9336134453781492, 2.8579831932773088, -0.17983193277311127, -2.2974789915966407, -1.1126050420168088, -0.5033613445378171, -1.3773109243697501, -1.2512605042016829, -0.10840336134453954, -1.730252100840338, 0.9630252100840311, 1.610084033613443, -0.8016806722689095, 3.1899159663865517, 5.34957983193277, 4.96302521008403, 3.0008403361344507, -0.1924369747899179, 0.15630252100840147, -0.25126050420168267, -1.1714285714285735, -0.17563025210084243, -0.2554621848739514, -1.4907563025210102, -2.5243697478991614, -0.2848739495798338, 0.20672268907562852, -2.68403361344538, -3.263865546218489, 0.07647058823529207, 4.231932773109242, 2.131092436974788, -0.7386554621848759, 0.30336134453781316, -0.818487394957985, -2.2134453781512624, -2.125210084033615, 0.017647058823527573, -0.33949579831932986, -1.0831932773109267, 1.3579831932773088, 2.7949579831932754, 0.5554621848739474, -1.8731092436974812]
  out "Off-Line  Bin Readings":dbl[](array[numeric])=[1588.0, 2151.0, 2569.0, 2952.0, 3024.0, 3012.0, 3039.0, 2811.0, 2726.0, 2533.0, 2508.0, 2309.0, 2206.0, 2059.0, 1874.0, 1901.0, 1639.0, 1756.0, 1566.0, 1578.0, 1429.0, 1420.0, 1400.0, 1361.0, 1293.0, 1186.0, 1183.0, 1138.0, 1181.0, 1096.0, 1114.0, 1130.0, 1077.0, 1010.0, 1026.0, 1029.0, 969.0, 956.0, 998.0, 988.0, 927.0, 923.0, 895.0, 898.0, 929.0, 912.0, 906.0, 877.0, 1112.0, 1264.0, 4424.0, 29160.0, 29305.0, 12628.0, 1004.0, 738.0, 755.0, 699.0, 701.0, 736.0, 704.0, 749.0, 740.0, 671.0, 651.0, 726.0, 674.0, 727.0, 774.0, 687.0, 708.0, 755.0, 709.0, 708.0, 748.0, 720.0, 730.0, 706.0, 732.0, 713.0, 753.0, 727.0, 702.0, 693.0, 735.0, 727.0, 730.0, 705.0, 687.0, 720.0, 715.0, 689.0, 682.0, 739.0, 729.0, 694.0, 649.0, 696.0, 722.0, 669.0, 716.0, 665.0, 640.0, 706.0, 700.0, 707.0, 729.0, 728.0, 674.0, 685.0, 651.0, 684.0, 719.0, 720.0, 717.0, 692.0, 712.0, 707.0, 741.0, 710.0, 681.0, 696.0, 761.0, 694.0, 678.0, 716.0, 699.0, 719.0, 688.0, 686.0, 692.0, 784.0, 718.0, 679.0, 755.0, 718.0, 715.0, 667.0, 742.0, 721.0, 716.0, 729.0, 747.0, 730.0, 708.0, 742.0, 724.0, 690.0, 748.0, 722.0, 719.0, 674.0, 706.0, 718.0, 710.0, 698.0, 763.0, 710.0, 685.0, 689.0, 644.0, 710.0, 688.0, 649.0, 730.0, 706.0, 704.0, 682.0, 690.0, 734.0, 721.0, 735.0, 668.0, 709.0, 679.0, 722.0, 679.0, 721.0, 726.0, 684.0, 712.0, 783.0, 721.0, 692.0, 720.0, 683.0, 756.0, 784.0, 725.0, 740.0, 713.0, 687.0, 682.0, 760.0, 736.0, 704.0, 680.0, 726.0, 727.0, 736.0, 723.0, 675.0, 680.0, 700.0, 714.0, 681.0, 744.0, 693.0, 660.0, 709.0, 669.0, 725.0, 696.0, 679.0, 664.0, 710.0, 711.0, 682.0, 677.0, 713.0, 732.0, 689.0, 729.0, 707.0, 704.0, 736.0, 708.0, 771.0, 720.0, 687.0, 685.0, 697.0, 756.0, 678.0, 747.0, 671.0, 702.0, 705.0, 755.0, 717.0, 763.0, 726.0, 670.0, 712.0, 733.0, 665.0, 682.0, 747.0, 767.0, 719.0, 714.0, 696.0, 746.0, 698.0, 698.0, 703.0, 731.0, 736.0, 719.0, 753.0, 702.0, 703.0, 740.0, 752.0, 654.0, 698.0, 708.0, 738.0, 731.0, 665.0, 746.0, 688.0, 666.0, 690.0, 698.0, 728.0, 712.0, 673.0, 754.0]
  out "Off-Line Smoothed":dbl[](array[numeric])=[1171.913846153846, 1693.6995604395613, 2111.1160439560454, 2391.2270329670346, 2554.4720879120905, 2596.1435164835193, 2524.0665934065955, 2374.476483516485, 2188.195164835166, 2012.5182417582423, 1857.318241758242, 1715.9918681318686, 1577.2358241758247, 1433.7523076923078, 1296.4424175824172, 1168.697362637362, 1051.6138461538449, 949.0149450549441, 858.8797802197794, 783.1006593406585, 720.1028571428562, 661.8391208791202, 609.3347252747247, 566.2303296703293, 525.76989010989, 487.89626373626356, 456.96439560439546, 428.60175824175803, 402.3435164835164, 379.3720879120878, 356.8534065934066, 335.0742857142857, 316.3632967032967, 298.00285714285735, 280.7138461538465, 267.0589010989014, 255.15890109890137, 243.352307692308, 232.44681318681347, 220.58967032967064, 210.53582417582442, 205.85230769230787, 205.69516483516503, 219.9545054945057, 266.43252747252757, 335.0731868131867, 397.190769230769, 461.7578021978019, 544.7490109890105, 700.4995604395596, 1540.517142857142, 2781.7874725274733, 5398.881978021976, 8117.967692307682, 7992.528131868121, 5383.030329670326, 2591.6863736263754, 1281.574285714286, 843.5830769230761, 936.3061538461527, 1249.273186813186, 1513.223736263736, 1672.7325274725276, 1778.5028571428572, 1745.9259340659341, 1574.011648351648, 1434.767692307692, 1346.96, 1188.7556043956042, 971.9797802197795, 859.9402197802192, 893.1435164835159, 901.576483516483, 818.588571428571, 639.7193406593403, 368.936923076923, 120.69076923076928, 8.212747252747244, -2.424615384615391, -2.4136263736263808, -1.1465934065934136, -1.6235164835164886, -3.4564835164835217, -3.293846153846161, -3.9839560439560495, -4.059780219780226, -3.514725274725282, -3.4982417582417655, -2.6839560439560515, -4.083956043956048, -4.932307692307695, -3.4191208791208854, -1.7685714285714356, -1.8575824175824247, -2.6927472527472602, -2.4246153846153917, -2.057582417582424, -1.921318681318688, -2.1158241758241827, -2.1696703296703364, -2.3663736263736337, -3.081758241758249, -3.730109890109897, -2.1652747252747315, -1.0751648351648417, -2.432307692307699, -1.1103296703296768, -0.7509890109890178, -3.9367032967033024, -3.1147252747252803, 0.6676923076923019, 5.802857142857141, 6.949010989010986, 3.586373626373621, 3.820439560439557, 13.217142857142829, 32.47318681318677, 47.47098901098897, 47.48087912087908, 36.931428571428526, 26.33362637362632, 15.743516483516462, 9.130329670329676, 10.641318681318683, 18.972087912087904, 33.889670329670295, 46.87978021978016, 52.36989010989004, 52.24241758241753, 48.497362637362585, 37.559999999999945, 24.536923076923024, 15.325934065934039, 7.877582417582421, 3.5028571428571413, 1.0325274725274658, -2.4037362637362705, -3.2356043956044025, -2.5927472527472593, -3.4718681318681393, -4.38285714285715, -3.1993406593406655, -2.2400000000000073, -2.2663736263736336, -2.5971428571428636, -2.619120879120886, -0.3345054945055011, -0.39054945054945706, -1.1257142857142923, -1.2817582417582485, -1.6927472527472596, -1.5059340659340723, -1.7718681318681386, -1.2345054945055014, -0.18835164835165488, -0.09054945054945715, -1.7136263736263806, -3.411428571428579, -1.6443956043956114, -0.1971428571428635, -1.175164835164842, -1.8696703296703365, -3.365274725274732, -4.223516483516491, -3.3927472527472595, -2.5465934065934133, -2.619120879120886, -1.010329670329677, 0.012747252747246085, -0.5301098901098966, 0.11054945054944415, -0.4575824175824241, -0.3400000000000066, -0.07626373626374289, -1.9960439560439633, -0.5246153846153923, 1.3391208791208722, -0.5213186813186879, -1.400439560439567, -1.0312087912087977, -0.9213186813186878, -1.1520879120879186, -0.8740659340659409, -0.3652747252747322, 0.501758241758235, -0.7246153846153917, -2.865274725274733, -1.07296703296704, 0.25670329670329034, -1.818021978021985, -2.094945054945062, -1.8630769230769302, -0.6520879120879193, -0.5191208791208868, -3.2575824175824253, -3.247692307692315, -0.4762637362637434, 1.2259340659340594, -0.6509890109890175, -0.7817582417582483, -0.47626373626374296, -1.3279120879120947, -1.0498901098901166, -1.3696703296703363, -0.3169230769230835, -0.6630769230769298, -1.422417582417589, 0.3303296703296642, 0.3226373626373564, -0.5158241758241825, -1.3641758241758308, -1.4652747252747318, -1.3257142857142923, -2.275164835164842, -1.3729670329670396, -1.0180219780219848, -1.7279120879120948, -0.46527472527473185, -0.8246153846153919, -1.9081318681318753, -0.7751648351648416, 0.10395604395603755, 0.024835164835158435, -0.2257142857142922, 1.5171428571428505, 2.2358241758241695, 0.006153846153839737, 0.9094505494505429, 1.444615384615378, -0.20703296703297358, 0.2336263736263672, 0.8457142857142792, -0.34329670329670986, -0.9400000000000064, -0.7301098901098965, -2.0356043956044023, -1.2542857142857213, 0.38637362637361994, -0.8806593406593469, -0.3707692307692372, 0.292967032967026, -1.1674725274725344, -1.8872527472527543, -1.2169230769230839, 0.07098901098900445, 0.06769230769230122, -0.1641758241758296, -0.25648351648352197, -0.3520879120879187, 0.5753846153846087, 0.9676923076923009, -0.10153846153846821, 0.21494505494504856, -0.47846153846154504, -1.4993406593406662, -1.0971428571428636, -1.0883516483516549, -1.040000000000006, -0.8476923076923139, -1.6125274725274796, -1.461978021978029, -0.845494505494512, -2.231208791208798, -0.7718681318681389, -0.14329670329670985, -1.6257142857142923, -1.0564835164835231, -0.2905494505494573, -0.8246153846153913, -2.383956043956051, 0.15010989010988296, 1.910549450549444, -2.3443956043956073, -1.2312087912087948, 2.892967032967025, 1.1314285714285643, -0.4158241758241824]
  out "On-Line  Smoothed":dbl[](array[numeric])=[1219.715824175825, 1697.7026373626384, 2060.879560439562, 2285.253186813188, 2393.3795604395614, 2385.8301098901106, 2266.961978021979, 2082.438901098902, 1876.5169230769234, 1685.66087912088, 1519.5257142857158, 1365.1773626373642, 1216.7531868131878, 1078.9520879120882, 951.5630769230773, 835.2400000000002, 734.6762637362639, 649.0378021978022, 574.4685714285713, 512.1872527472525, 460.5883516483515, 415.9586813186811, 376.26967032966996, 341.3367032967029, 311.05978021978, 283.5465934065933, 258.8751648351647, 237.27846153846139, 217.80043956043943, 200.14329670329664, 186.14109890109887, 172.5389010989011, 157.38285714285718, 146.05648351648358, 137.57626373626383, 128.0685714285715, 119.54219780219785, 111.59054945054947, 102.52021978021983, 96.74000000000008, 93.31692307692317, 89.3389010989012, 88.09934065934077, 95.56747252747257, 116.31582417582416, 145.67406593406594, 170.93890109890106, 193.5399999999999, 223.93780219780214, 287.2619780219779, 694.7191208791206, 1281.196043956044, 2468.542197802197, 3679.8685714285684, 3391.6509890109865, 2092.3817582417582, 961.3641758241766, 454.629010989011, 306.4641758241754, 356.10703296703264, 483.3751648351647, 577.8476923076923, 626.3927472527473, 658.9784615384615, 635.8290109890108, 560.8312087912086, 504.43120879120846, 469.77516483516445, 408.4147252747249, 326.36967032967016, 288.55868131868124, 303.5509890109888, 301.8345054945054, 272.629010989011, 212.08835164835165, 111.99494505494508, 30.375164835164846, 1.9993406593406622, -1.9720879120879093, -2.7270329670329643, -1.6127472527472506, -1.1435164835164813, -0.7226373626373609, -2.062197802197799, -3.002857142857139, -3.2182417582417555, -3.677582417582414, -3.025934065934063, -3.1512087912087874, -2.9116483516483482, -1.6292307692307668, -1.5808791208791186, -1.341318681318679, -2.002857142857141, -1.1797802197802183, -1.0676923076923062, -2.550109890109888, -2.5149450549450525, -1.4336263736263715, -0.5149450549450533, -0.5589010989010972, -2.561098901098899, -3.1380219780219756, -1.6753846153846137, -2.667692307692305, -2.7446153846153822, -1.6676923076923056, -1.9940659340659321, -0.8589010989010971, 0.011428571428573397, 0.38725274725274916, 2.1037362637362667, 1.4136263736263766, -1.1501098901098878, 1.1784615384615402, 5.813626373626378, 10.783956043956046, 14.155384615384612, 13.1454945054945, 10.83010989010989, 7.143296703296709, 4.674065934065938, 2.6279120879120916, 1.9674725274725322, 5.175164835164839, 10.36857142857143, 15.433406593406595, 14.494945054945056, 12.86527472527472, 13.110329670329664, 9.67736263736264, 6.15098901098902, 2.1246153846153915, 0.39604395604395837, -0.1391208791208769, -0.9742857142857123, -0.4654945054945034, -1.6083516483516456, -0.9149450549450523, -0.26329670329670163, -0.9149450549450531, -0.661098901098899, -1.3314285714285694, -1.3632967032967014, -0.7589010989010971, -0.48527472527472343, 1.8191208791208815, 0.633406593406596, -2.209450549450547, -0.26769230769230556, 0.15428571428571636, -0.5292307692307673, 0.6806593406593423, 0.5894505494505511, 0.44879120879121054, -0.1951648351648334, -1.2632967032967017, -1.268791208791207, -1.6149450549450526, -1.4468131868131846, -0.9270329670329653, -3.2863736263736247, -3.5654945054945038, -0.1610989010988994, 0.4015384615384634, 0.2454945054945075, -1.8391208791208762, -2.505054945054942, -1.5479120879120867, -1.707252747252746, -2.7610989010988973, -2.9479120879120844, -1.0731868131868116, -0.27318681318681143, 0.21032967032967204, -0.9632967032967011, -0.2094505494505473, -0.17758241758241577, -2.189670329670328, -1.5138461538461523, 0.7542857142857159, 0.43230769230769406, -1.1797802197802176, 0.8070329670329693, 1.7773626373626394, -0.180879120879119, -1.4204395604395579, -0.8753846153846129, -0.4259340659340641, -0.2072527472527454, -0.20175824175823992, -1.9039560439560417, -1.6797802197802176, -0.745714285714284, -1.1270329670329653, -0.15890109890109716, 0.5169230769230786, -1.023736263736262, -0.8512087912087893, -0.19186813186812995, -0.7248351648351627, -0.7775824175824156, 0.5586813186813208, 1.3378021978021999, 0.18725274725274899, -0.6786813186813169, -1.0973626373626355, -0.8094505494505475, -0.5391208791208777, -0.6182417582417568, -1.4270329670329651, -1.1885714285714268, 0.5136263736263755, 0.9235164835164855, -0.6852747252747236, -1.9358241758241732, -3.6149450549450513, -3.781978021978019, -0.7248351648351625, 0.8213186813186832, -0.22593406593406434, -1.150109890109888, -0.5830769230769208, 0.1729670329670347, -0.46659340659340476, -0.7490109890109872, 0.4015384615384633, 0.15098901098901285, -0.8391208791208773, 0.46087912087912275, 0.010329670329672136, -0.290769230769229, 1.0158241758241775, 0.7916483516483535, 1.2696703296703316, 1.869670329670332, 0.6520879120879145, -1.035824175824174, 0.9553846153846178, 2.054285714285717, 0.22791208791208986, -0.18307692307692122, -1.4665934065934048, -1.40175824175824, -1.9358241758241737, -1.3742857142857123, 0.08615384615384791, -0.02263736263736088, 1.8542857142857159, 2.3367032967032983, 0.987252747252749, -0.3116483516483499, -0.27758241758241575, 0.1674725274725292, 0.04769230769230929, 0.5257142857142875, 0.13120879120879309, 0.2400000000000017, 1.4806593406593422, 1.2125274725274746, 0.650989010989013, -0.37978021978021803, -0.368791208791207, 0.19274725274725457, 0.16637362637362818, 0.5520879120879139, 0.49384615384615554, 0.9982417582417595, 0.32571428571428707, -0.2995604395604377, -0.09406593406593211, 0.04769230769230953, 0.5938461538461557, -0.1984615384615366, -0.3171428571428553, -0.1830769230769212, 0.11252747252747441]
  out "On-Line Bin Readings":dbl[](array[numeric])=[1605.0, 2079.0, 2519.0, 2803.0, 2900.0, 2869.0, 2823.0, 2778.0, 2484.0, 2313.0, 2021.0, 1933.0, 1844.0, 1653.0, 1598.0, 1464.0, 1411.0, 1372.0, 1317.0, 1279.0, 1127.0, 1097.0, 1059.0, 1033.0, 994.0, 961.0, 912.0, 897.0, 895.0, 831.0, 909.0, 836.0, 849.0, 886.0, 831.0, 800.0, 856.0, 841.0, 784.0, 815.0, 755.0, 814.0, 768.0, 773.0, 741.0, 768.0, 776.0, 788.0, 848.0, 870.0, 2394.0, 15105.0, 14110.0, 4247.0, 761.0, 661.0, 715.0, 685.0, 689.0, 699.0, 710.0, 736.0, 668.0, 676.0, 737.0, 693.0, 742.0, 668.0, 675.0, 692.0, 713.0, 697.0, 687.0, 715.0, 707.0, 670.0, 677.0, 695.0, 775.0, 662.0, 679.0, 721.0, 674.0, 671.0, 719.0, 704.0, 659.0, 684.0, 680.0, 688.0, 679.0, 750.0, 712.0, 704.0, 728.0, 708.0, 688.0, 713.0, 680.0, 708.0, 715.0, 667.0, 698.0, 684.0, 712.0, 664.0, 674.0, 701.0, 707.0, 677.0, 674.0, 716.0, 714.0, 731.0, 629.0, 706.0, 659.0, 712.0, 694.0, 674.0, 701.0, 680.0, 663.0, 660.0, 741.0, 693.0, 690.0, 678.0, 661.0, 654.0, 650.0, 684.0, 681.0, 703.0, 698.0, 707.0, 670.0, 701.0, 688.0, 675.0, 745.0, 695.0, 703.0, 730.0, 728.0, 682.0, 692.0, 692.0, 693.0, 764.0, 665.0, 712.0, 714.0, 700.0, 687.0, 734.0, 722.0, 740.0, 692.0, 719.0, 732.0, 711.0, 649.0, 690.0, 644.0, 700.0, 637.0, 714.0, 686.0, 669.0, 714.0, 670.0, 695.0, 692.0, 678.0, 702.0, 652.0, 747.0, 693.0, 713.0, 675.0, 725.0, 682.0, 671.0, 672.0, 630.0, 686.0, 706.0, 693.0, 721.0, 684.0, 733.0, 729.0, 682.0, 664.0, 718.0, 705.0, 681.0, 688.0, 647.0, 673.0, 671.0, 706.0, 679.0, 721.0, 662.0, 656.0, 690.0, 680.0, 652.0, 689.0, 690.0, 735.0, 629.0, 673.0, 702.0, 679.0, 706.0, 689.0, 706.0, 738.0, 698.0, 673.0, 661.0, 698.0, 672.0, 702.0, 706.0, 684.0, 736.0, 697.0, 671.0, 717.0, 694.0, 696.0, 660.0, 709.0, 688.0, 730.0, 713.0, 755.0, 728.0, 701.0, 678.0, 710.0, 666.0, 709.0, 698.0, 669.0, 675.0, 685.0, 737.0, 689.0, 695.0, 681.0, 704.0, 664.0, 682.0, 700.0, 663.0, 740.0, 684.0, 718.0, 739.0, 684.0, 704.0, 669.0, 716.0, 676.0, 707.0, 719.0, 668.0, 718.0, 726.0, 641.0, 630.0, 685.0, 723.0, 739.0]
  out "Range Corrected Altitude Array":dbl[](array[numeric])=[5625.0, 22500.0, 50625.0, 90000.0, 140625.0, 202500.0, 275625.0, 360000.0, 455625.0, 562500.0, 680625.0, 810000.0, 950625.0, 1102500.0, 1265625.0, 1440000.0, 1625625.0, 1822500.0, 2030625.0, 2250000.0, 2480625.0, 2722500.0, 2975625.0, 3240000.0, 3515625.0, 3802500.0, 4100625.0, 4410000.0, 4730625.0, 5062500.0, 5405625.0, 5760000.0, 6125625.0, 6502500.0, 6890625.0, 7290000.0, 7700625.0, 8122500.0, 8555625.0, 9000000.0, 9455625.0, 9922500.0, 10400625.0, 10890000.0, 11390625.0, 11902500.0, 12425625.0, 12960000.0, 13505625.0, 14062500.0, 14630625.0, 15210000.0, 15800625.0, 16402500.0, 17015625.0, 17640000.0, 18275625.0, 18922500.0, 19580625.0, 20250000.0, 20930625.0, 21622500.0, 22325625.0, 23040000.0, 23765625.0, 24502500.0, 25250625.0, 26010000.0, 26780625.0, 27562500.0, 28355625.0, 29160000.0, 29975625.0, 30802500.0, 31640625.0, 32490000.0, 33350625.0, 34222500.0, 35105625.0, 36000000.0, 36905625.0, 37822500.0, 38750625.0, 39690000.0, 40640625.0, 41602500.0, 42575625.0, 43560000.0, 44555625.0, 45562500.0, 46580625.0, 47610000.0, 48650625.0, 49702500.0, 50765625.0, 51840000.0, 52925625.0, 54022500.0, 55130625.0, 56250000.0, 57380625.0, 58522500.0, 59675625.0, 60840000.0, 62015625.0, 63202500.0, 64400625.0, 65610000.0, 66830625.0, 68062500.0, 69305625.0, 70560000.0, 71825625.0, 73102500.0, 74390625.0, 75690000.0, 77000625.0, 78322500.0, 79655625.0, 81000000.0, 82355625.0, 83722500.0, 85100625.0, 86490000.0, 87890625.0, 89302500.0, 90725625.0, 92160000.0, 93605625.0, 95062500.0, 96530625.0, 98010000.0, 99500625.0, 101002500.0, 102515625.0, 104040000.0, 105575625.0, 107122500.0, 108680625.0, 110250000.0, 111830625.0, 113422500.0, 115025625.0, 116640000.0, 118265625.0, 119902500.0, 121550625.0, 123210000.0, 124880625.0, 126562500.0, 128255625.0, 129960000.0, 131675625.0, 133402500.0, 135140625.0, 136890000.0, 138650625.0, 140422500.0, 142205625.0, 144000000.0, 145805625.0, 147622500.0, 149450625.0, 151290000.0, 153140625.0, 155002500.0, 156875625.0, 158760000.0, 160655625.0, 162562500.0, 164480625.0, 166410000.0, 168350625.0, 170302500.0, 172265625.0, 174240000.0, 176225625.0, 178222500.0, 180230625.0, 182250000.0, 184280625.0, 186322500.0, 188375625.0, 190440000.0, 192515625.0, 194602500.0, 196700625.0, 198810000.0, 200930625.0, 203062500.0, 205205625.0, 207360000.0, 209525625.0, 211702500.0, 213890625.0, 216090000.0, 218300625.0, 220522500.0, 222755625.0, 225000000.0, 227255625.0, 229522500.0, 231800625.0, 234090000.0, 236390625.0, 238702500.0, 241025625.0, 243360000.0, 245705625.0, 248062500.0, 250430625.0, 252810000.0, 255200625.0, 257602500.0, 260015625.0, 262440000.0, 264875625.0, 267322500.0, 269780625.0, 272250000.0, 274730625.0, 277222500.0, 279725625.0, 282240000.0, 284765625.0, 287302500.0, 289850625.0, 292410000.0, 294980625.0, 297562500.0, 300155625.0, 302760000.0, 305375625.0, 308002500.0, 310640625.0, 313290000.0, 315950625.0, 318622500.0, 321305625.0, 324000000.0, 326705625.0, 329422500.0, 332150625.0, 334890000.0, 337640625.0, 340402500.0, 343175625.0, 345960000.0, 348755625.0, 351562500.0, 354380625.0, 357210000.0, 360050625.0, 362902500.0, 365765625.0, 368640000.0, 371525625.0, 374422500.0, 377330625.0, 380250000.0, 383180625.0, 386122500.0, 389075625.0, 392040000.0, 395015625.0, 398002500.0, 401000625.0, 404010000.0, 407030625.0, 410062500.0, 413105625.0, 416160000.0, 419225625.0, 422302500.0, 425390625.0, 428490000.0, 431600625.0, 434722500.0, 437855625.0, 441000000.0]
  out "Altitude Array (km)":dbl[](array[numeric])=[0.075, 0.15, 0.22499999999999998, 0.3, 0.375, 0.45, 0.5249999999999999, 0.6, 0.6749999999999999, 0.7499999999999999, 0.825, 0.8999999999999999, 0.9749999999999999, 1.05, 1.125, 1.2, 1.275, 1.3499999999999999, 1.4249999999999998, 1.5, 1.575, 1.65, 1.7249999999999999, 1.7999999999999998, 1.8749999999999998, 1.95, 2.025, 2.1, 2.1750000000000003, 2.25, 2.325, 2.4, 2.475, 2.5500000000000003, 2.625, 2.7, 2.775, 2.85, 2.9250000000000003, 3.0, 3.075, 3.15, 3.225, 3.3000000000000003, 3.375, 3.45, 3.525, 3.6, 3.675, 3.75, 3.825, 3.9, 3.975, 4.05, 4.125, 4.2, 4.275, 4.35, 4.425, 4.5, 4.575, 4.65, 4.725, 4.8, 4.875, 4.95, 5.025, 5.1, 5.175, 5.25, 5.325, 5.4, 5.475, 5.55, 5.625, 5.7, 5.775, 5.85, 5.925, 6.0, 6.075, 6.15, 6.225, 6.3, 6.375, 6.45, 6.525, 6.6, 6.675, 6.75, 6.825, 6.9, 6.975, 7.05, 7.125, 7.2, 7.2749999999999995, 7.35, 7.425, 7.5, 7.575, 7.6499999999999995, 7.725, 7.8, 7.875, 7.95, 8.024999999999999, 8.1, 8.174999999999999, 8.249999999999998, 8.325, 8.399999999999999, 8.475, 8.549999999999999, 8.624999999999998, 8.7, 8.774999999999999, 8.85, 8.924999999999999, 8.999999999999998, 9.075, 9.149999999999999, 9.225, 9.299999999999999, 9.374999999999998, 9.45, 9.524999999999999, 9.6, 9.674999999999999, 9.749999999999998, 9.825, 9.899999999999999, 9.975, 10.049999999999999, 10.124999999999998, 10.2, 10.274999999999999, 10.35, 10.424999999999999, 10.499999999999998, 10.575, 10.649999999999999, 10.725, 10.799999999999999, 10.874999999999998, 10.95, 11.024999999999999, 11.1, 11.174999999999999, 11.249999999999998, 11.325, 11.399999999999999, 11.475, 11.549999999999999, 11.624999999999998, 11.7, 11.774999999999999, 11.85, 11.924999999999999, 11.999999999999998, 12.075, 12.149999999999999, 12.225, 12.299999999999999, 12.374999999999998, 12.45, 12.524999999999999, 12.6, 12.674999999999999, 12.749999999999998, 12.825, 12.899999999999999, 12.975, 13.049999999999999, 13.124999999999998, 13.2, 13.274999999999999, 13.35, 13.424999999999999, 13.499999999999998, 13.575, 13.649999999999999, 13.725, 13.799999999999999, 13.874999999999998, 13.95, 14.024999999999999, 14.1, 14.174999999999999, 14.249999999999998, 14.325, 14.399999999999999, 14.474999999999998, 14.549999999999999, 14.624999999999998, 14.7, 14.774999999999999, 14.849999999999998, 14.924999999999999, 14.999999999999998, 15.075, 15.149999999999999, 15.224999999999998, 15.299999999999999, 15.374999999999998, 15.45, 15.524999999999999, 15.599999999999998, 15.674999999999999, 15.749999999999998, 15.825, 15.899999999999999, 15.974999999999998, 16.05, 16.125, 16.2, 16.275, 16.349999999999998, 16.424999999999997, 16.5, 16.575, 16.65, 16.724999999999998, 16.799999999999997, 16.875, 16.95, 17.025, 17.099999999999998, 17.174999999999997, 17.25, 17.325, 17.4, 17.474999999999998, 17.549999999999997, 17.625, 17.7, 17.775, 17.849999999999998, 17.924999999999997, 18.0, 18.075, 18.15, 18.224999999999998, 18.299999999999997, 18.375, 18.45, 18.525, 18.599999999999998, 18.674999999999997, 18.75, 18.825, 18.9, 18.974999999999998, 19.049999999999997, 19.125, 19.2, 19.275, 19.349999999999998, 19.424999999999997, 19.5, 19.575, 19.65, 19.724999999999998, 19.799999999999997, 19.875, 19.95, 20.025, 20.099999999999998, 20.174999999999997, 20.25, 20.325, 20.4, 20.474999999999998, 20.549999999999997, 20.625, 20.7, 20.775, 20.849999999999998, 20.924999999999997, 21.0]
  out "Offline Pulse Energy":dbl=4.689372857142857
  out "Online Pulse Energy":dbl=4.70368
  in  "Instrument Control":T5(tab)=enum."Wavemeter"
  in  "ILX Address On":dbl=1.0 min=0.0 step=1.0
  in  "ILX Address Off":dbl=2.0 min=0.0 step=1.0
  in  "OnLineLD":dbl=169.7
  in  "OffLineLD":dbl=172.62
  in  "Pulse B Polarity":enum32{"Low", "High"}(ring)=enum."High"
  in  "Pulse A Delay(ns)":u32=1040 min=80 max=327600
  in  "Pulse B Delay(ns)":u32=170000 min=80 max=327600 step=1
  in  "Accumulation Delay(ns)":u32=10 min=10 max=1270 step=1
  in  "Sync Pulse Polarity":enum32{"Low", "High"}(ring)=enum."High"
  in  "Pulse A Polarity":enum32{"Low", "High"}(ring)=enum."High"
  in  "Number of Bins":u32=280 min=2 max=4095 step=1
  in  "Number of Accumulates":u32=10000 min=1 max=32767 step=1
  in  "Time Resolution Per Bin(ns)":u32=500 min=5 max=1063 step=1
  in  "Lambda On Set (nm)":dbl=828.198 format="%.5f"
  out "Lambda On Read (nm)":dbl=828.1979602252092 format="%.5f"
  out "Lambda Off Read (nm)":dbl=828.2976895457859 format="%.5f"
  in  "Lambda Off Set (nm)":dbl=828.29765 format="%#.5f"
  in  "Bristol In":i32=5
  out "Bristol Out":i32
  out "WL_Difference":dbl=-3.9774790820956696e-05 format="%#_3e"
  out "WL Difference off":dbl=3.9545785966765834e-05 format="%#_3e"
  out "Wavelength Lock Online":bool=TRUE
  out "Wavelength Lock Offline":bool=TRUE
  in  "calculate absorption cross sections":bool
  in  "Online_Tol":dbl=5e-05 format="%#_15g"
  in  "Cancel online":bool
  in  "Offline_Tol":dbl=5e-05 format="%#_15g"
  in  "Smoothing Range":dbl=150.0
  in  "Total DIAL Integration Time (Minutes)":i32=3
  in  "Data Reads (number of loops)":i32=1
  in  "Total Aerosol Integration Time (Minutes)":dbl=0.5
  in  "Scalar Wait Time":u32
  out "Smoothed Bins":dbl=2.0
  in  "NewportIn":string
  in  "logging":bool
  out "Newport Device Key":string="1918-R 15120"
  in  "SampleSize":i32=2
  out "NewportRef":refnum<k24>
  in  "Switch Comm Port":refnum<visa-resource-name>="COM3"
  out "FF_On_Ref":refnum<file>
  out "FF_On_Ptr":i64=4422704 format="%.2p"
  out "FF_Off_Ref":refnum<file>
  out "FF_Off_Ptr":i64=4422704 format="%.2p"
  out "NF_On_Ref":refnum<file>
  out "NF_On_Ptr":i64=4422704 format="%.2p"
  out "NF_Off_Ref":refnum<file>
  out "NF_Off_Ptr":i64=4422704 format="%.2p"
  out "DataOpen":bool=TRUE
  out "File Path_Far Field (out)":string="C:\\Users\\H2ODial\\Desktop\\SharedTeleWVData\\160815FF\\21"
  out "File Path_Near Field (out)":string="C:\\Users\\H2ODial\\Desktop\\SharedTeleWVData\\160815NF\\21"
  in  "Data File DIR (in)":string="C:\\Users\\H2ODial\\Desktop\\SharedTeleWVData\\"
  in  "bins":u32=280 min=2 max=4095 step=1
  out "y offset":u32=10
  in  "ns scale":u32=500
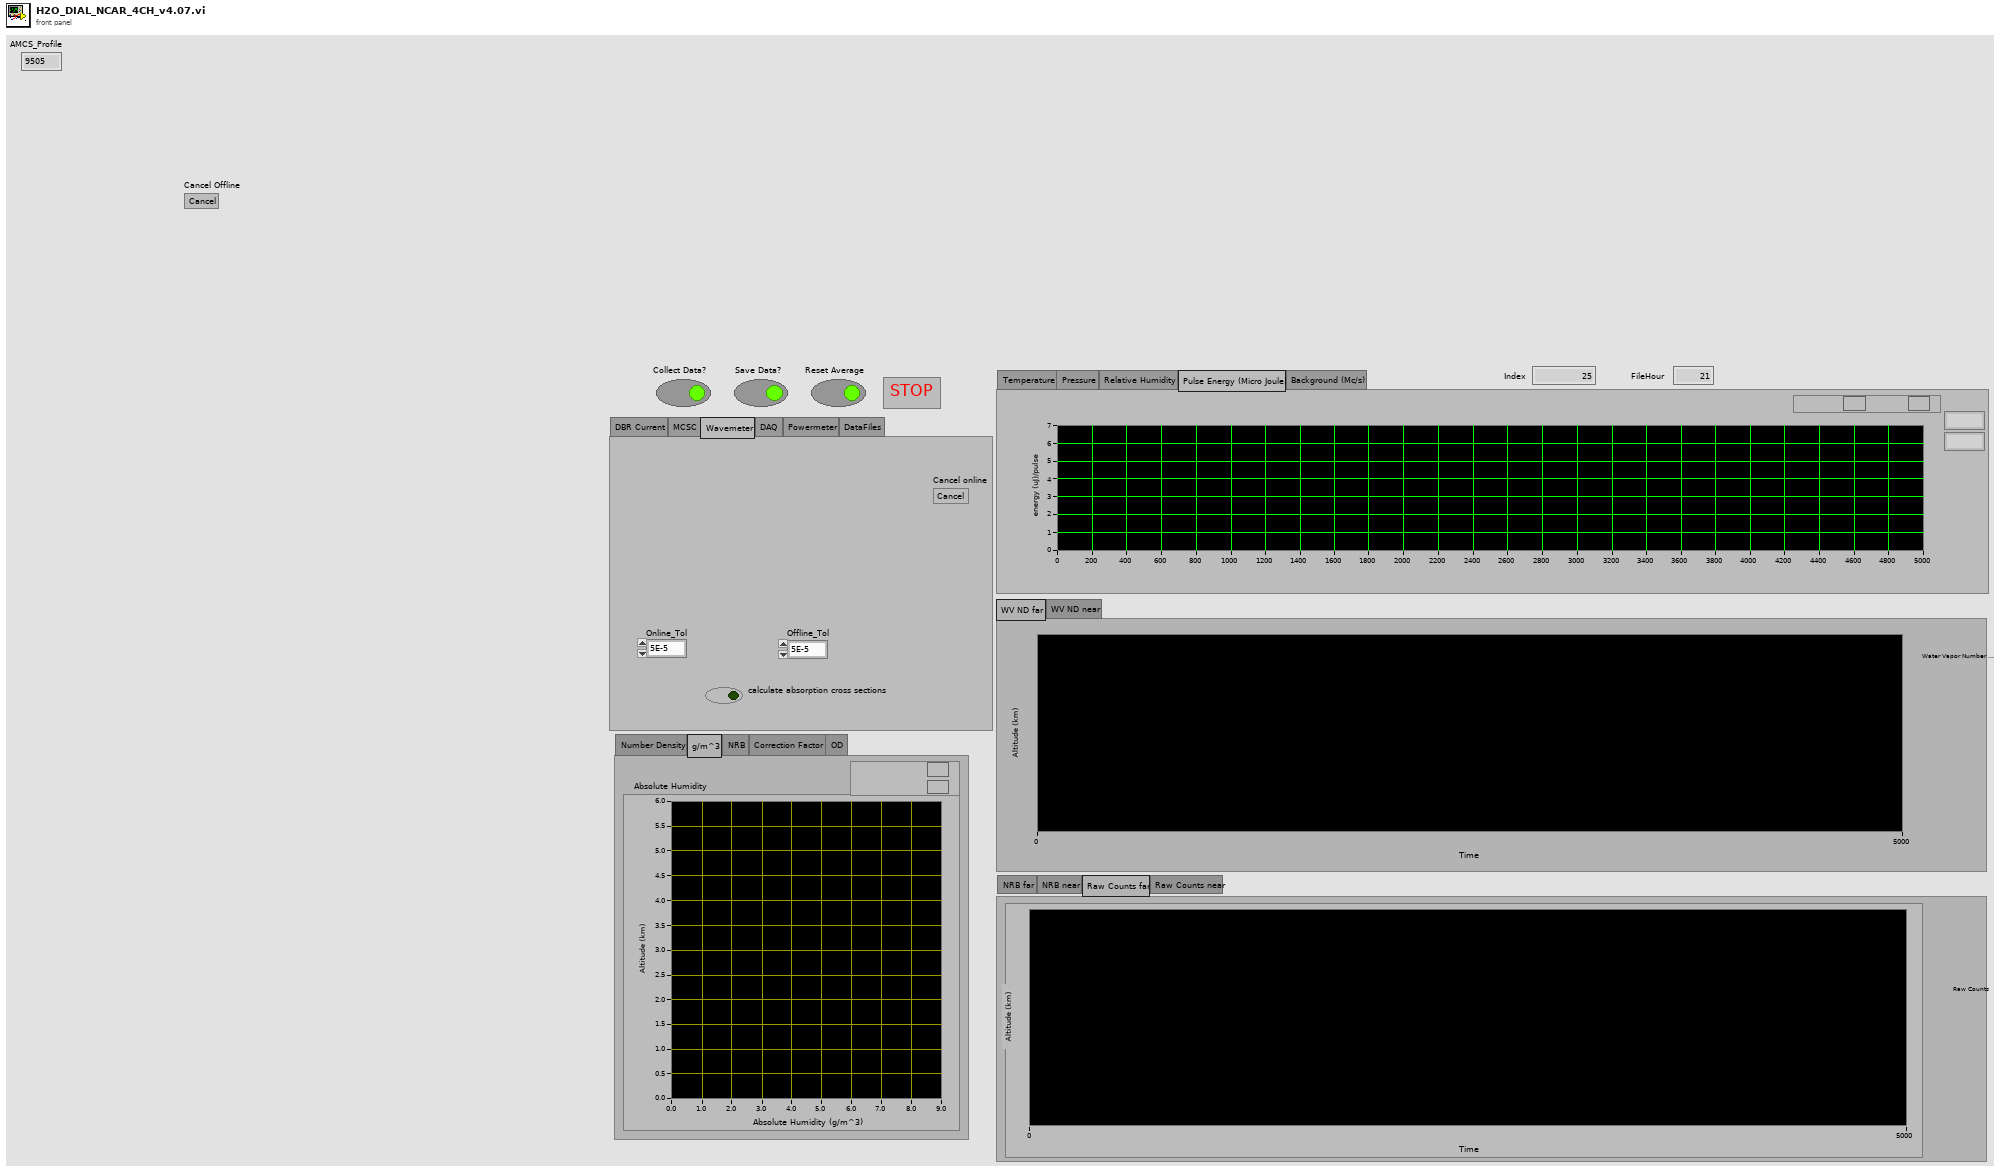
[diagram p1: front panel]
types:
  T1 = enum32{"NRB far", "NRB near", "Raw Counts far", "Raw Counts near"}
  T2 = enum32{"Number Density", "g/m^3", "NRB", "Correction Factor", "OD"}
  T3 = enum32{"Temperature", "Pressure", "Relative Humidity", "Pulse Energy (Micro Joule)", "Background (Mc/s)"}
  T4 = cluster{"Online Pulse Energy":dbl, "Pulse Energy Offline":dbl}
  T5 = enum32{"DBR Current", "MCSC", "Wavemeter", "DAQ", "Powermeter", "DataFiles"}
  T6 = enum16{"Initialize ILX", "Set ON T", "Set Off T", "Set ON I", "Set Off I", "Set On Lim", "Set Off Lim", "Read ILX", "TEC ON/OFF", "LASER ON/OFF", "Status?", "ILX OFF"}
  T7 = enum16{"open", "replace", "create", "open or create", "replace or create", "replace or create with confirmation"}
  T8 = typedef "LVDateTimeRec.ctl" = cluster{"fractional second":dbl, "second":i32, "minute":i32, "hour":i32, "day of month":i32, "month":i32, "year":i32, "day of week":i32, "day of year":i32, "DST":i32}
  T9 = cluster{"Online Pulse Energy":dbl, "Offline Pulse Energy":dbl}
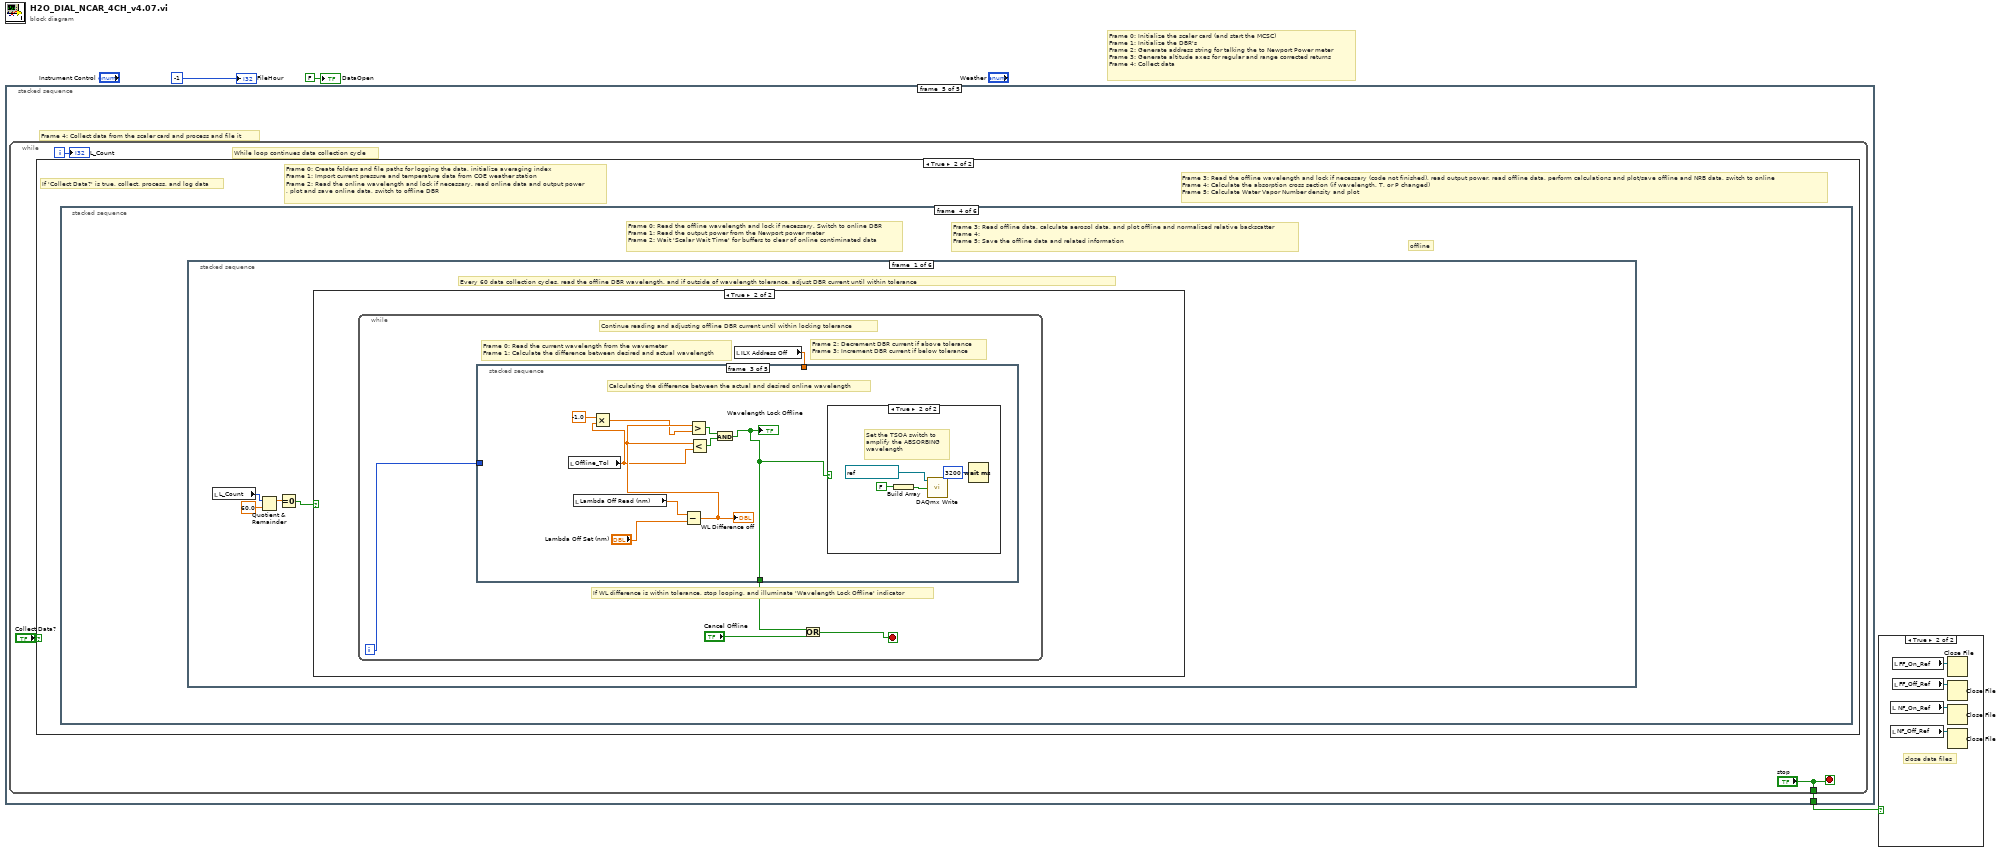
[diagram p0: block diagram]
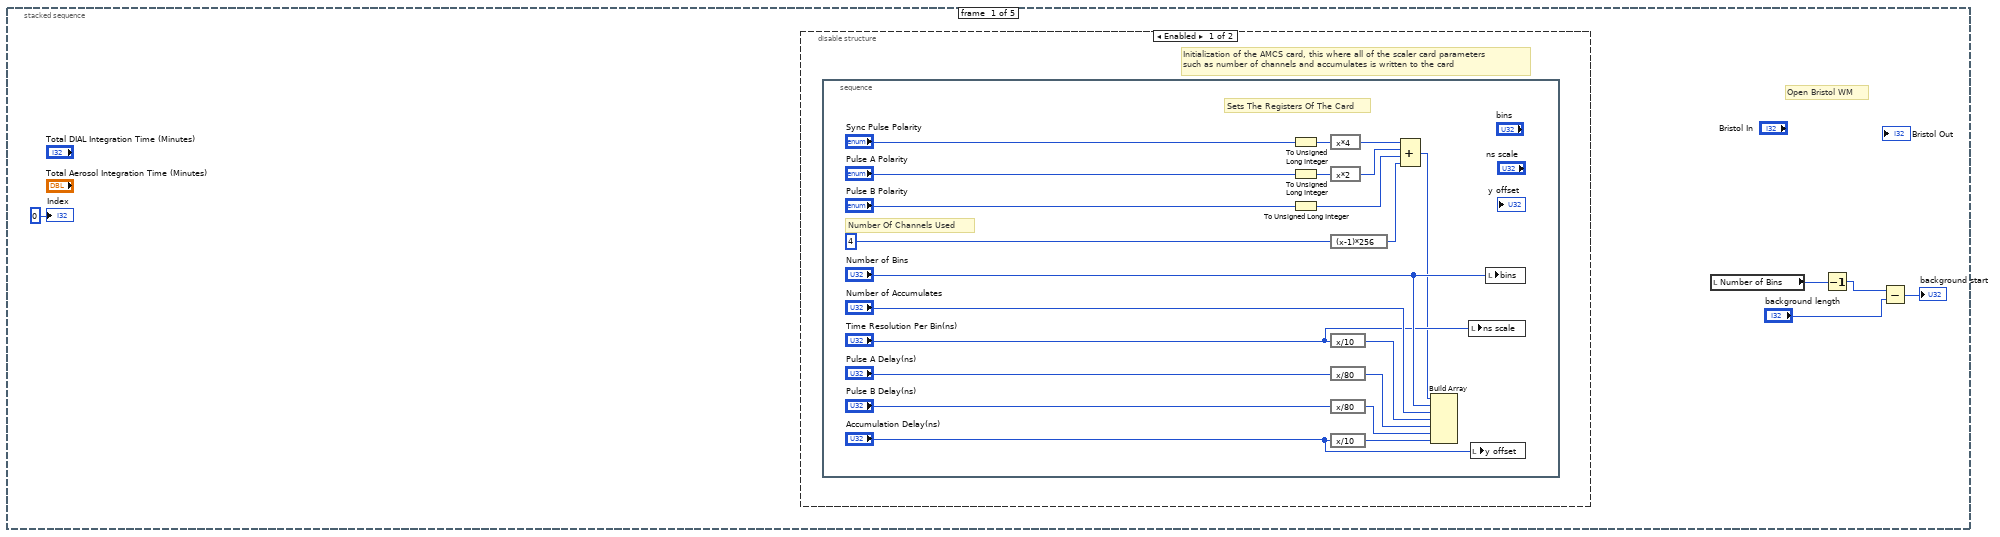
[diagram p3: hidden frame]
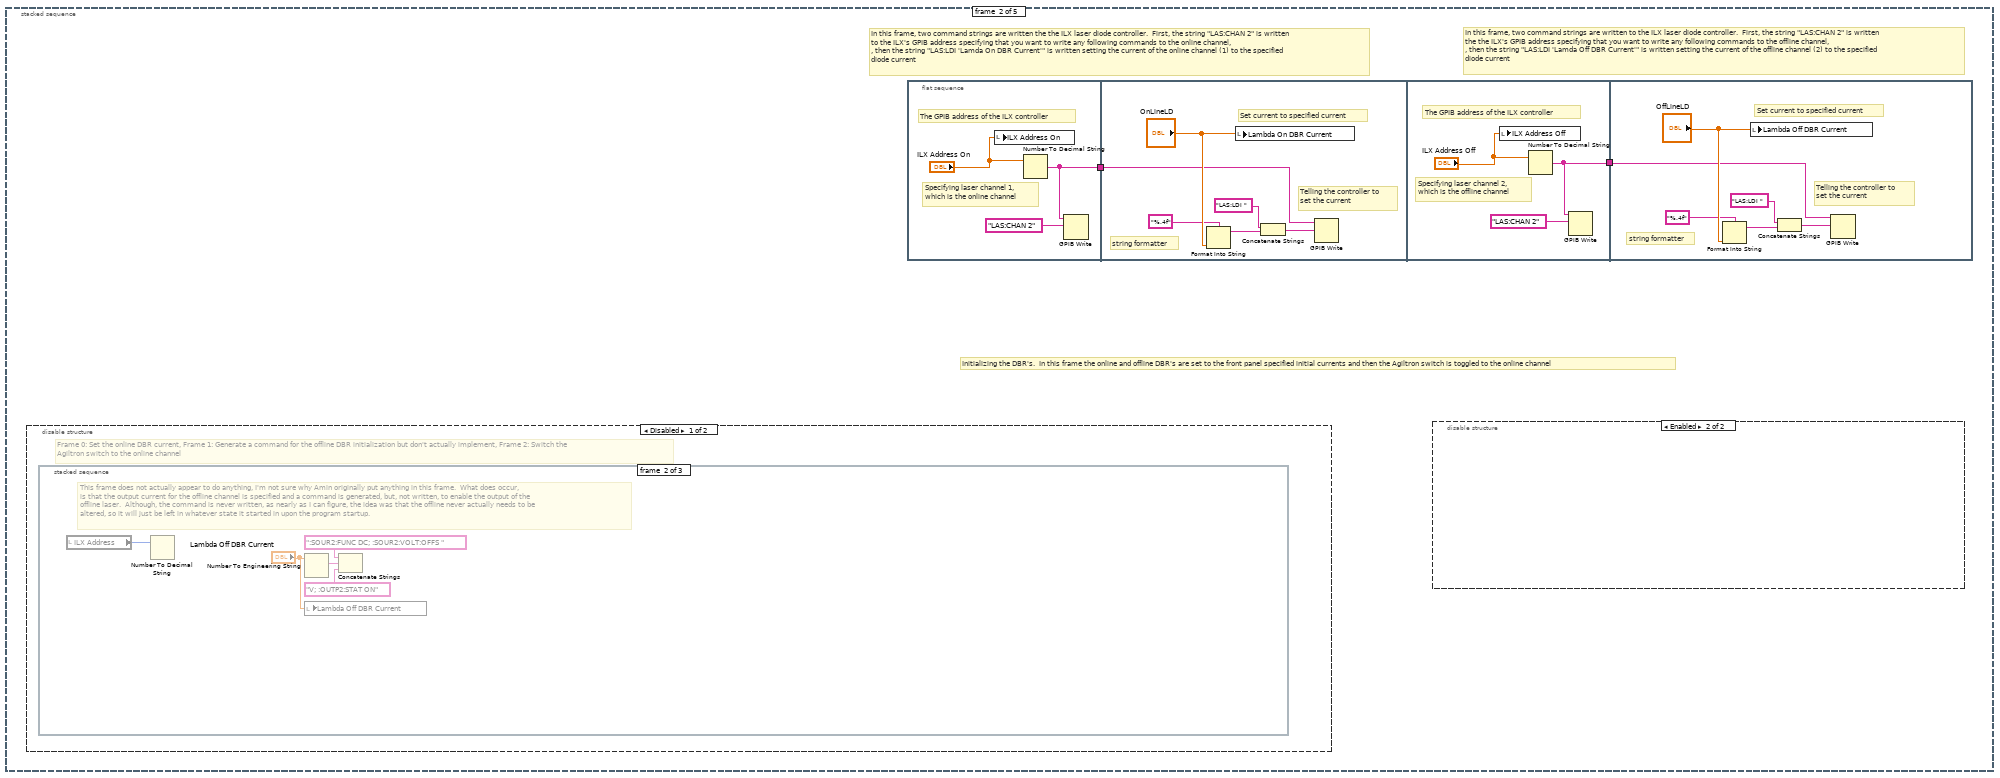
[diagram p5: hidden frame]
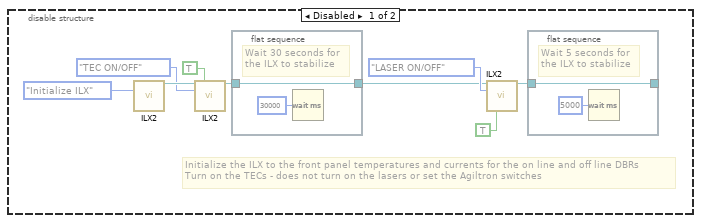
[diagram p6: hidden frame]
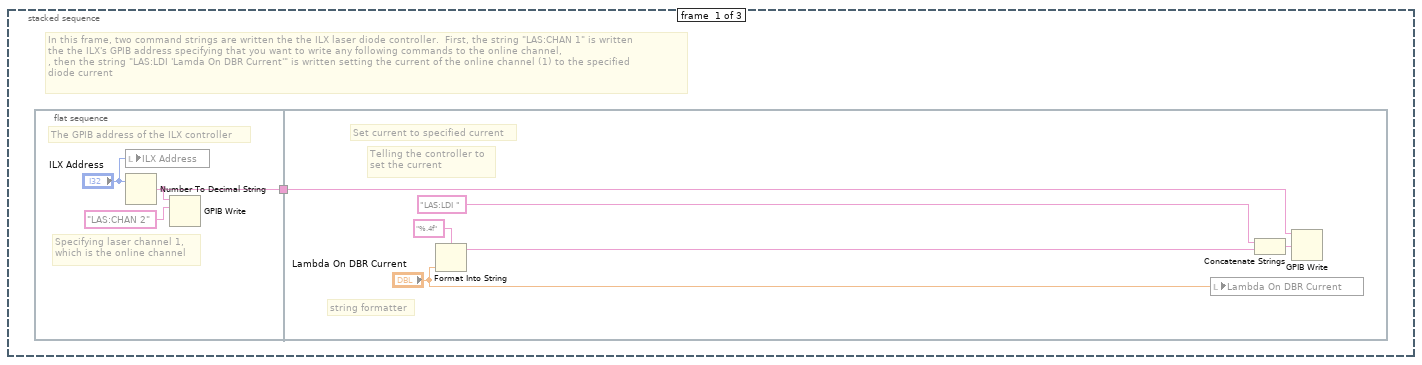
[diagram p7: hidden frame]
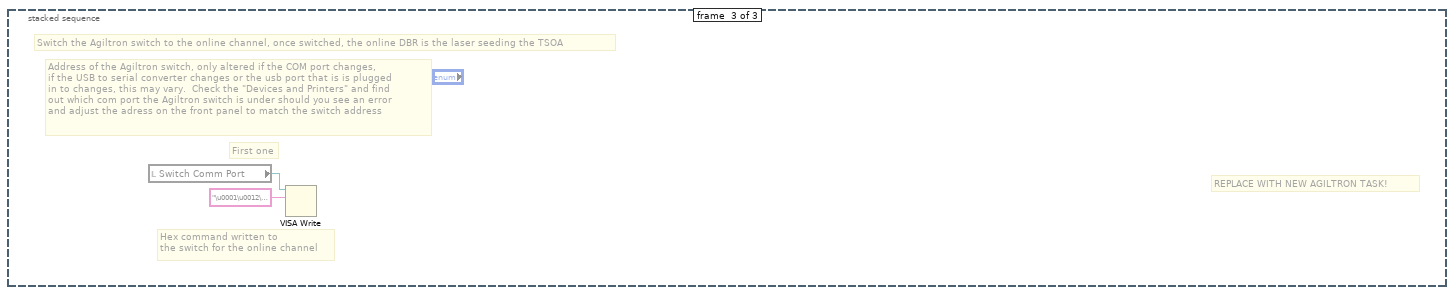
[diagram p8: hidden frame]
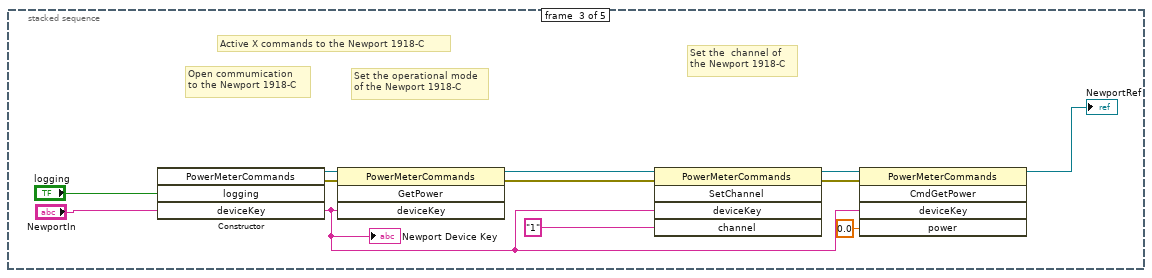
[diagram p10: hidden frame]
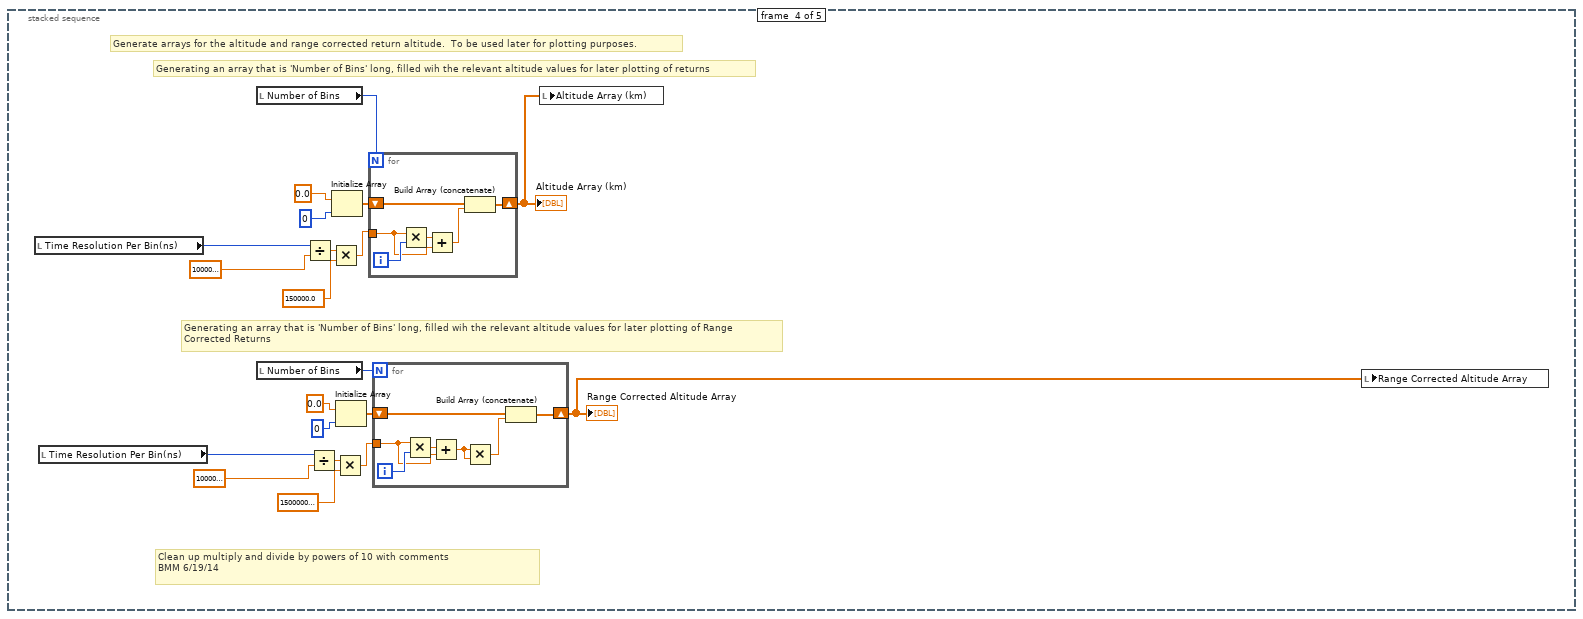
[diagram p11: hidden frame]
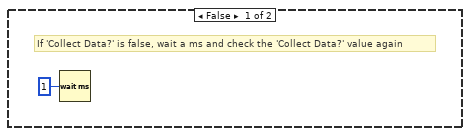
[diagram p12: hidden frame]
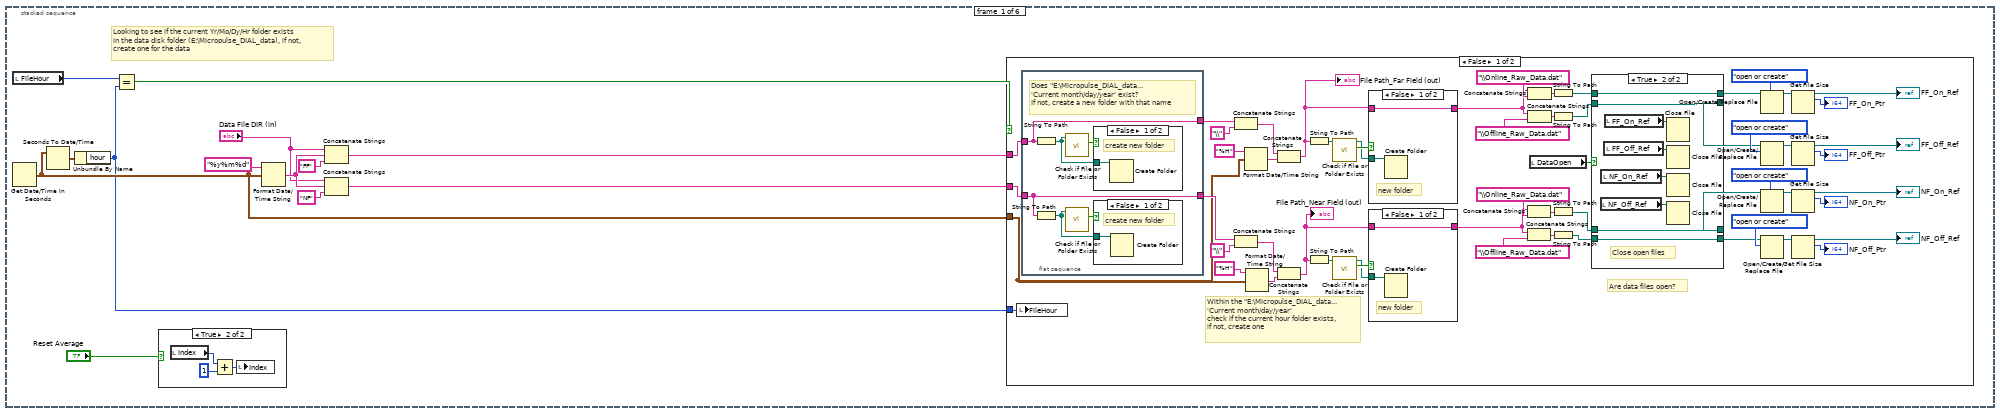
[diagram p13: hidden frame]
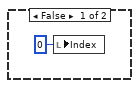
[diagram p20: hidden frame]
diagram:
  # "Frame 0: Initialize the scaler card (and start the MCSC)\nFrame 1: Initialize the DBR's\nFrame 2: Generate address string for talking the to Newport Power meter\nFrame 3: Generate altitude axes for regular and range corrected returns\nFrame 4: Collect data"
  n1 = stacked-sequence {
    tunnel: [_ _ _ _ w125] -> w3
    frame #0 {
      # "Open Bristol WM"
      n2 = disable-structure shown="Enabled" {
        frame Enabled {
          # "Initialization of the AMCS card, this where all of the scaler card parameters\nsuch as number of channels and accumulates is written to the card"
          n3 = stacked-sequence {
            frame #0 {
              # "Sets The Registers Of The Card"
              # "Number Of Channels Used"
              n4 = To Unsigned Long Integer(number="Sync Pulse Polarity") -> (unsigned 32bit integer=w9:u32)
              n5 = To Unsigned Long Integer(number="Pulse A Polarity") -> (unsigned 32bit integer=w13:u32)
              n6 = To Unsigned Long Integer(number="Pulse B Polarity") -> (unsigned 32bit integer=w11:u32)
              n7 = expression code="x*4"(w9) -> (w18:u32)
              n8 = expression code="x*2"(w13) -> (w17:u32)
              n9 = expression code="(x-1)*256"(u32 4 ("Number of Channels Used")) -> (w16:u32)
              n10 = expression code="x/10"("Time Resolution Per Bin(ns)") -> (w20:u32)
              n11 = expression code="x/80"("Pulse A Delay(ns)") -> (w27:u32)
              n12 = expression code="x/80"("Pulse B Delay(ns)") -> (w29:u32)
              n13 = expression code="x/10"("Accumulation Delay(ns)") -> (w28:u32)
              n14 = Compound Arithmetic op=ADD(w18, w17, w11, w16) -> (w15:u32)
              n15 = Build Array(w15, "Number of Bins", "Number of Accumulates", w20, w27, w29, w28) -> ()  [unwired: 1 out]
              n16 = local write "ns scale"("Time Resolution Per Bin(ns)") -> ()
              n17 = local write "y offset"("Accumulation Delay(ns)") -> ()
              n18 = local write "bins"("Number of Bins") -> ()
            }
          }
        }
        frame Disabled {
        }
      }
      n19 = local read "Number of Bins"() -> (w7:u32)
      n20 = Decrement(x=w7) -> (x-1=w6:u32)
      n21 = Subtract(x=w6, y="background length") -> (x-y=→"background start":u32)
      "Index" <- 0 ("Index")
    }
    frame #1 {
      # "In this frame, two command strings are written to the ILX laser diode controller.  First, the string \"LAS:CHAN 2\" is written\nthe the ILX's GPIB address specifying that you want to write any following commands to the offline channel,\n, then the string \"LAS:LDI 'Lamda Off DBR Current'\" is written setting the current of the offline channel (2) to the specified \ndiode current"
      # "In this frame, two command strings are written the the ILX laser diode controller.  First, the string \"LAS:CHAN 2\" is written\nto the ILX's GPIB address specifying that you want to write any following commands to the online channel,\n, then the string \"LAS:LDI 'Lamda On DBR Current'\" is written setting the current of the online channel (1) to the specified \ndiode current"
      # "Initializing the DBR's.  In this frame the online and offline DBR's are set to the front panel specified initial currents and then the Agiltron switch is toggled to the online channel"
      n22 = disable-structure shown="Disabled" {
        frame Disabled {
          # "Frame 0: Set the online DBR current, Frame 1: Generate a command for the offline DBR initialization but don't actually implement, Frame 2: Switch the \nAgiltron switch to the online channel"
          n23 = stacked-sequence {
            frame #0 {
              # "In this frame, two command strings are written the the ILX laser diode controller.  First, the string \"LAS:CHAN 1\" is written\nthe the ILX's GPIB address specifying that you want to write any following commands to the online channel,\n, then the string \"LAS:LDI 'Lamda On DBR Current'\" is written setting the current of the online channel (1) to the specified \ndiode current"
              n24 = flat-sequence {
                tunnel: [w65] -> w63
                tunnel: w63 -> [w67]
                frame #0 {
                  # "The GPIB address of the ILX controller"
                  # "Specifying laser channel 1,\nwhich is the online channel"
                  n25 = local write "ILX Address"("ILX Address") -> ()
                  n26 = Number To Decimal String(number="ILX Address") -> (decimal integer string=w65:string)  [unwired: 1 in]
                  n27 = GPIB Write(0:w65, 1:"LAS:CHAN 2") -> ()  [unwired: 3 in, 2 out]
                }
                frame #1 {
                  # "Telling the controller to\nset the current"
                  # "string formatter"
                  # "Set current to specified current"
                  n28 = Format Into String(format string="%.4f" ("Format String"), "Lambda On DBR Current") -> (resulting string=w70:string)  [unwired: 2 in, 1 out]
                  n29 = local write "Lambda On DBR Current"("Lambda On DBR Current") -> ()
                  n30 = Concatenate Strings("LAS:LDI ", w70) -> (w71:string)
                  n31 = GPIB Write(0:w67, 1:w71) -> ()  [unwired: 3 in, 2 out]
                }
              }
            }
            frame #1 {
              # "This frame does not actually appear to do anything, I'm not sure why Amin originally put anything in this frame.  What does occur, \nis that the output current for the offline channel is specified and a command is generated, but, not written, to enable the output of the\noffline laser.  Although, the command is never written, as nearly as I can figure, the idea was that the offline never actually needs to be \naltered, so it will just be left in whatever state it started in upon the program startup."
              n32 = local read "ILX Address"() -> (w73:i32)
              n33 = Number To Decimal String(number=w73) -> ()  [unwired: 1 in, 1 out]
              n34 = Number To Engineering String(4:"Lambda Off DBR Current") -> (0:w77:string)  [unwired: 3 in]
              n35 = local write "Lambda Off DBR Current"("Lambda Off DBR Current") -> ()
              n36 = Concatenate Strings(":SOUR2:FUNC DC; :SOUR2:VOLT:OFFS ", w77, "V; :OUTP2:STAT ON") -> ()  [unwired: 1 out]
            }
            frame #2 {
              # "REPLACE WITH NEW AGILTRON TASK!"
              # "First one"
              # "Address of the Agiltron switch, only altered if the COM port changes,\nif the USB to serial converter changes or the usb port that is is plugged\nin to changes, this may vary.  Check the \"Devices and Printers\" and find \nout which com port the Agiltron switch is under should you see an error \nand adjust the adress on the front panel to match the switch address"
              # "Hex command written to \nthe switch for the online channel"
              # "Switch the Agiltron switch to the online channel, once switched, the online DBR is the laser seeding the TSOA"
              n37 = local read "Switch Comm Port"() -> (w78:refnum<visa-resource-name>)
              n38 = VISA Write(VISA resource name=w78, write buffer="\u0001\u0012\u0000\u0002") -> ()  [unwired: 1 in, 3 out]
            }
          }
        }
        frame Enabled {
        }
      }
      n39 = flat-sequence {
        tunnel: [w33] -> w31
        tunnel: w31 -> [w35]
        tunnel: [w41] -> w30
        tunnel: w30 -> [w44]
        frame #0 {
          # "The GPIB address of the ILX controller"
          # "Specifying laser channel 1,\nwhich is the online channel"
          n40 = local write "ILX Address On"("ILX Address On") -> ()
          n41 = Number To Decimal String(number="ILX Address On") -> (decimal integer string=w33:string)  [unwired: 1 in]
          n42 = GPIB Write(0:w33, 1:"LAS:CHAN 2") -> ()  [unwired: 3 in, 2 out]
        }
        frame #1 {
          # "Telling the controller to\nset the current"
          # "string formatter"
          # "Set current to specified current"
          n43 = Format Into String(format string="%.4f" ("Format String"), "OnLineLD") -> (resulting string=w38:string)  [unwired: 2 in, 1 out]
          n44 = local write "Lambda On DBR Current"("OnLineLD") -> ()
          n45 = Concatenate Strings("LAS:LDI ", w38) -> (w39:string)
          n46 = GPIB Write(0:w35, 1:w39) -> ()  [unwired: 3 in, 2 out]
        }
        frame #2 {
          # "The GPIB address of the ILX controller"
          # "Specifying laser channel 2,\nwhich is the offline channel"
          n47 = local write "ILX Address Off"("ILX Address Off") -> ()
          n48 = Number To Decimal String(number="ILX Address Off") -> (decimal integer string=w41:string)  [unwired: 1 in]
          n49 = GPIB Write(0:w41, 1:"LAS:CHAN 2") -> ()  [unwired: 3 in, 2 out]
        }
        frame #3 {
          # "Telling the controller to\nset the current"
          # "string formatter"
          # "Set current to specified current"
          n50 = Format Into String(format string="%.4f" ("Format String"), "OffLineLD") -> (resulting string=w47:string)  [unwired: 2 in, 1 out]
          n51 = local write "Lambda Off DBR Current"("OffLineLD") -> ()
          n52 = Concatenate Strings("LAS:LDI ", w47) -> (w48:string)
          n53 = GPIB Write(0:w44, 1:w48) -> ()  [unwired: 3 in, 2 out]
        }
      }
      n54 = disable-structure shown="Enabled" {
        frame Disabled {
          # "Initialize the ILX to the front panel temperatures and currents for the on line and off line DBRs\nTurn on the TECs - does not turn on the lasers or set the Agiltron switches"
          n55 = call "ILX2.vi"("ILX Command"=T6."Initialize ILX") -> ("Device Out"=w57:refnum<visa-resource-name>)  [unwired: 10 in, 4 out]
          n56 = call "ILX2.vi"("Device In"=w57, "TEC Control"=TRUE, "ILX Command"=T6."TEC ON/OFF") -> ("Device Out"=w54:refnum<visa-resource-name>)  [unwired: 8 in, 4 out]
          n57 = flat-sequence {
            tunnel: w54 -> [w61]
            tunnel: [w61] -> w51
            frame #0 {
              # "Wait 30 seconds for\nthe ILX to stabilize"
              n58 = Wait (ms)(milliseconds to wait=u32 30000) -> ()  [unwired: 1 out]
            }
          }
          n59 = call "ILX2.vi"("Device In"=w51, "ILX Command"=T6."LASER ON/OFF", "Laser Control"=TRUE ("TEC Control")) -> ("Device Out"=w50:refnum<visa-resource-name>)  [unwired: 8 in, 4 out]
          n60 = flat-sequence {
            tunnel: w50 -> [w59]
            tunnel: [w59] -> _
            frame #0 {
              # "Wait 5 seconds for\nthe ILX to stabilize"
              n61 = Wait (ms)(milliseconds to wait=u32 5000) -> ()  [unwired: 1 out]
            }
          }
        }
        frame Enabled {
        }
      }
    }
    frame #2 {
      # "Active X commands to the Newport 1918-C"
      # "Set the  channel of\nthe Newport 1918-C"
      # "Set the operational mode\nof the Newport 1918-C"
      # "Open commumication\nto the Newport 1918-C"
      n62 = constructor class="PowerMeterCommands"("logging"="logging", "deviceKey"="NewportIn") -> (reference out=w91:refnum<k24>, error out=w88:errorcluster, "deviceKey"=w83:string)  [unwired: 3 in, 2 out]
      "Newport Device Key" <- w83
      n63 = invoke class="PowerMeterCommands" method="GetPower"(reference=w91, error in=w88, "deviceKey"=w83) -> (reference out=w90:refnum<k24>, error out=w87:errorcluster)  [unwired: 1 in, 2 out]
      n64 = invoke class="PowerMeterCommands" method="SetChannel"(reference=w90, error in=w87, "deviceKey"=w83, "channel"="1") -> (reference out=w84:refnum<k24>, error out=w86:errorcluster)  [unwired: 1 in, 3 out]
      n65 = invoke class="PowerMeterCommands" method="CmdGetPower"(reference=w84, error in=w86, "deviceKey"=w83, "power"=sgl 0.0) -> (reference out=→"NewportRef":refnum<k24>)  [unwired: 1 in, 4 out]
    }
    frame #3 {
      # "Clean up multiply and divide by powers of 10 with comments\nBMM 6/19/14"
      # "Generating an array that is 'Number of Bins' long, filled wih the relevant altitude values for later plotting of Range \nCorrected Returns"
      # "Generating an array that is 'Number of Bins' long, filled wih the relevant altitude values for later plotting of returns"
      # "Generate arrays for the altitude and range corrected return altitude.  To be used later for plotting purposes."
      n66 = local read "Time Resolution Per Bin(ns)"() -> (w104:u32)
      n67 = local read "Time Resolution Per Bin(ns)"() -> (w94:u32)
      n68 = local read "Number of Bins"() -> (w107:u32)
      n69 = local read "Number of Bins"() -> (w97:u32)
      n70 = Divide(x=w104, y=1000000000.0) -> (x/y=w102:dbl)
      n71 = Divide(x=w94, y=1000000000.0) -> (x/y=w92:dbl)
      n72 = Multiply(x=w102, y=150000.0) -> (x*y=w105:dbl)
      n73 = Initialize Array(0.0, 0) -> (w110:dbl[])
      n74 = Multiply(x=w92, y=150000000.0) -> (x*y=w95:dbl)
      n75 = Initialize Array(0.0, 0) -> (w100:dbl[])
      n76 = for {
        N: w107 -> [_]
        shift-right: [w123] -> w108
        shift-left: w110 -> [w124]
        tunnel: w105 -> [w120]
        i -> [w122]
        n77 = Multiply(x=w120, y=w122) -> (x*y=w121:dbl)
        n78 = Add(x=w121, y=w120) -> (x+y=w119:dbl)
        n79 = Build Array (concatenate)(w124, w119) -> (w123:dbl[])
      }
      "Altitude Array (km)" <- w108
      n80 = for {
        N: w97 -> [_]
        shift-right: [w117] -> w98
        shift-left: w100 -> [w118]
        tunnel: w95 -> [w113]
        i -> [w116]
        n81 = Multiply(x=w113, y=w116) -> (x*y=w114:dbl)
        n82 = Add(x=w114, y=w113) -> (x+y=w112:dbl)
        n83 = Multiply(x=w112, y=w112) -> (x*y=w115:dbl)
        n84 = Build Array (concatenate)(w118, w115) -> (w117:dbl[])
      }
      "Range Corrected Altitude Array" <- w98
      n85 = local write "Altitude Array (km)"(w108) -> ()
      n86 = local write "Range Corrected Altitude Array"(w98) -> ()
    }
    frame #4 {
      # "Frame 4: Collect data from the scaler card and process and file it"
      n87 = while {
        tunnel: ["stop"] -> w125
        i -> [w126]
        stop <- "stop" stop-if-true
        # "While loop continues data collection cycle"
        n88 = case shown="True" "Collect Data?" {
          frame False {
            # "If 'Collect Data?' is false, wait a ms and check the 'Collect Data?' value again"
            n89 = Wait (ms)(milliseconds to wait=u32 1) -> ()  [unwired: 1 out]
          }
          frame True {
            # "Frame 3: Read the offline wavelength and lock if necessary (code not finished), read output power, read offline data, perform calculations and plot/save offline and NRB data, switch to online\nFrame 4: Calculate the absorption cross section (if wavelength, T, or P changed)\nFrame 5: Calculate Water Vapor Number density and plot"
            # "Frame 0: Create folders and file paths for logging the data, initialize averaging index\nFrame 1: Import current pressure and temperature data from COE weather station\nFrame 2: Read the online wavelength and lock if necessary, read online data and output power\n, plot and save online data, switch to offline DBR"
            # "If 'Collect Data?' is true, collect, process, and log data"
            n90 = stacked-sequence {
              frame #0 {
                # "Looking to see if the current Yr/Mo/Dy/Hr folder exists\nin the data disk folder (E:\\Micropulse_DIAL_data), if not,\ncreate one for the data"
                n91 = local read "FileHour"() -> (w139:i32)
                n92 = Get Date/Time In Seconds() -> (seconds since 1Jan1904=w131:timestamp)
                n93 = Seconds To Date/Time(time stamp (now)=w131) -> (date time rec=w141:T8)  [unwired: 1 in]
                n94 = Unbundle By Name(w141) -> ("hour"=w130:i32)
                n95 = Equal?(x=w139, y=w130) -> (x = y?=w140:bool)
                n96 = case shown="True" "Reset Average" {
                  frame False {
                    n97 = local write "Index"(0 ("Index")) -> ()
                  }
                  frame True {
                    n98 = local read "Index"() -> (w229:i32)
                    n99 = Add(x=w229, y=1) -> (x+y=w228:i32)
                    n100 = local write "Index"(w228) -> ()
                  }
                }
                n101 = Format Date/Time String(time format string (%c)="%y%m%d", seconds (now)=w131) -> (date/time string=w135:string)  [unwired: 1 in]
                n102 = Concatenate Strings("Data File DIR (in)", w135, "FF" ("string")) -> (w137:string)
                n103 = Concatenate Strings("Data File DIR (in)", w135, "NF" ("string")) -> (w132:string)
                n104 = case shown="False" w140 {
                  tunnel: w137 -> [w199 _]
                  tunnel: w132 -> [w198 _]
                  tunnel: w131 -> [w185 _]
                  tunnel: w130 -> [w161 _]
                  frame False {
                    # "Are data files open?"
                    # "Within the \"E:\\Micropulse_DIAL_data...\n'Current month/day/year' \ncheck if the current hour folder exists,\nif not, create one"
                    n105 = local write "FileHour"(w161) -> ()
                    n106 = flat-sequence {
                      tunnel: [w219] -> w186
                      tunnel: w199 -> [w218]
                      tunnel: w198 -> [w219]
                      tunnel: [w218] -> w187
                      frame #0 {
                        # "Does \"E:\\Micropulse_DIAL_data...\n'Current month/day/year' exist?\nIf not, create a new folder with that name"
                        n107 = String To Path(string=w218) -> (path=w223:path)
                        n108 = String To Path(string=w219) -> (path=w221:path)
                        n109 = call <vilib>:"Check if File or Folder Exists.vi"("path"=w223) -> ("file or folder exists?"=w222:bool)  [unwired: 8 in, 2 out]
                        n110 = call <vilib>:"Check if File or Folder Exists.vi"("path"=w221) -> ("file or folder exists?"=w220:bool)  [unwired: 8 in, 2 out]
                        n111 = case shown="False" w222 {
                          tunnel: w223 -> [w225 _]
                          frame False {
                            # "create new folder"
                            n112 = Create Folder(path (use dialog)=w225) -> ()  [unwired: 2 in, 3 out]
                          }
                          frame True {
                            # "Folder exists\ndo nothing"
                          }
                        }
                        n113 = case shown="False" w220 {
                          tunnel: w221 -> [w224 _]
                          frame False {
                            # "create new folder"
                            n114 = Create Folder(path (use dialog)=w224) -> ()  [unwired: 2 in, 3 out]
                          }
                          frame True {
                            # "Folder exists\ndo nothing"
                          }
                        }
                      }
                    }
                    n115 = Concatenate Strings(w187, "\\" ("string")) -> (w194:string)
                    n116 = Concatenate Strings(w186, "\\" ("string")) -> (w189:string)
                    n117 = Format Date/Time String(time format string (%c)="%H", seconds (now)=w185) -> (date/time string=w197:string)  [unwired: 1 in]
                    n118 = Format Date/Time String(time format string (%c)="%H", seconds (now)=w185) -> (date/time string=w192:string)  [unwired: 1 in]
                    n119 = Concatenate Strings(w194, w197) -> (w157:string)
                    "File Path_Far Field (out)" <- w157
                    n120 = Concatenate Strings(w189, w192) -> (w158:string)
                    "File Path_Near Field (out)" <- w158
                    n121 = String To Path(string=w157) -> (path=w195:path)
                    n122 = String To Path(string=w158) -> (path=w190:path)
                    n123 = call <vilib>:"Check if File or Folder Exists.vi"("path"=w195) -> ("file or folder exists?"=w184:bool, "dup path"=w182:path)  [unwired: 8 in, 1 out]
                    n124 = call <vilib>:"Check if File or Folder Exists.vi"("path"=w190) -> ("file or folder exists?"=w183:bool, "dup path"=w181:path)  [unwired: 8 in, 1 out]
                    n125 = case shown="False" w184 {
                      tunnel: w182 -> [w216 _]
                      tunnel: w157 -> [w215 w217]
                      tunnel: [w215 w217] -> w155
                      frame False {
                        # "new folder"
                        n126 = Create Folder(path (use dialog)=w216) -> ()  [unwired: 2 in, 3 out]
                      }
                      frame True {
                        # "Folder exists\ndo nothing"
                      }
                    }
                    n127 = case shown="False" w183 {
                      tunnel: w181 -> [w213 _]
                      tunnel: w158 -> [w212 w214]
                      tunnel: [w212 w214] -> w156
                      frame False {
                        # "new folder"
                        n128 = Create Folder(path (use dialog)=w213) -> ()  [unwired: 2 in, 3 out]
                      }
                      frame True {
                        # "Folder exists\ndo nothing"
                      }
                    }
                    n129 = Concatenate Strings(w156, "\\Online_Raw_Data.dat" ("string")) -> (w175:string)
                    n130 = Concatenate Strings(w156, "\\Offline_Raw_Data.dat" ("string")) -> (w174:string)
                    n131 = Concatenate Strings(w155, "\\Online_Raw_Data.dat" ("string")) -> (w180:string)
                    n132 = Concatenate Strings(w155, "\\Offline_Raw_Data.dat" ("string")) -> (w179:string)
                    n133 = local read "DataOpen"() -> (w172:bool)
                    n134 = String To Path(string=w180) -> (path=w171:path)
                    n135 = String To Path(string=w179) -> (path=w170:path)
                    n136 = String To Path(string=w175) -> (path=w169:path)
                    n137 = String To Path(string=w174) -> (path=w168:path)
                    n138 = case shown="True" w172 {
                      tunnel: w171 -> [w203 w207]
                      tunnel: [w203 w207] -> w165
                      tunnel: w170 -> [w202 w206]
                      tunnel: [w202 w206] -> w164
                      tunnel: w169 -> [w201 w205]
                      tunnel: [w201 w205] -> w163
                      tunnel: [w200 w204] -> w162
                      tunnel: w168 -> [w200 w204]
                      frame False {
                        # "No files open\ndo nothing"
                      }
                      frame True {
                        # "Close open files"
                        n139 = local read "NF_Off_Ref"() -> (w209:refnum<file>)
                        n140 = local read "NF_On_Ref"() -> (w208:refnum<file>)
                        n141 = local read "FF_Off_Ref"() -> (w211:refnum<file>)
                        n142 = local read "FF_On_Ref"() -> (w210:refnum<file>)
                        n143 = Close File(refnum=w210) -> ()  [unwired: 1 in, 2 out]
                        n144 = Close File(refnum=w211) -> ()  [unwired: 1 in, 2 out]
                        n145 = Close File(refnum=w208) -> ()  [unwired: 1 in, 2 out]
                        n146 = Close File(refnum=w209) -> ()  [unwired: 1 in, 2 out]
                      }
                    }
                    n147 = Open/Create/Replace File(file path (use dialog)=w165, operation (0:open)=T7."open or create") -> (refnum out=w151:refnum<file>)  [unwired: 4 in, 2 out]
                    n148 = Open/Create/Replace File(file path (use dialog)=w164, operation (0:open)=T7."open or create") -> (refnum out=w152:refnum<file>)  [unwired: 4 in, 2 out]
                    n149 = Open/Create/Replace File(file path (use dialog)=w163, operation (0:open)=T7."open or create") -> (refnum out=w153:refnum<file>)  [unwired: 4 in, 2 out]
                    n150 = Open/Create/Replace File(file path (use dialog)=w162, operation (0:open)=T7."open or create") -> (refnum out=w154:refnum<file>)  [unwired: 4 in, 2 out]
                    n151 = Get File Size(file=w151) -> (refnum out=→"FF_On_Ref":refnum<file>, size (in bytes)=→"FF_On_Ptr":i64)  [unwired: 1 in, 1 out]
                    n152 = Get File Size(file=w152) -> (refnum out=→"FF_Off_Ref":refnum<file>, size (in bytes)=→"FF_Off_Ptr":i64)  [unwired: 1 in, 1 out]
                    n153 = Get File Size(file=w153) -> (refnum out=→"NF_On_Ref":refnum<file>, size (in bytes)=→"NF_On_Ptr":i64)  [unwired: 1 in, 1 out]
                    n154 = Get File Size(file=w154) -> (refnum out=→"NF_Off_Ref":refnum<file>, size (in bytes)=→"NF_Off_Ptr":i64)  [unwired: 1 in, 1 out]
                  }
                  frame True {
                    # "Don't need to do anything!"
                  }
                }
              }
              frame #1 {
                # "Writing and plotting retrieved\nweather parameters"
                # "Matlab script goes online and retrieves most recent press, temp, and relative humidity data \nfrom the weather station on the roof of Cobleigh"
                # "Importing the current weather conditions from the COE weather station"
                n155 = disable-structure shown="Disabled" {
                  frame Disabled {
                    n156 = script code="%try\n%s=urlread('http://www.coe.montana.edu/ee/weather/mostCurrentCSV.php');\n%amin=textscan(s,'%s %s %s %s %s %s %s %s %s %s %s %s %s');\n%data=amin{1}{2};\n%[test remain]=strtok(data,',');\n%remain=str2num(remain);\n%press=remain(3)./1000;\n%temp=remain(5);\n%RH=remain(7);\n%catch\npress=.850;\ntemp=20;\nRH=40;\n%end"() -> ()  [unwired: 1 in, 4 out]
                  }
                  frame Enabled {
                  }
                }
                "Temperature (C)" <- "Temperature (C)"
                "Pressure (mb)" <- "Pressure (mbar or hPa)"
                "Relative Humdity (%)" <- 40.0 ("Real")
              }
              frame #2 {
                # "Frame 3: Read, process, and plot online data\nFrame 4:\nFrame 5: Write the data to the folders from Frame 0 of outter sequence"
                # "Frame 0: Read the online wavelength and adjust to locking tolerance if out of range, Switch to offline DBR\nFrame 1: Read the output power from the Newport meter, calculate and plot the output pulse energy\nFrame 2: Wait 'Scalar Wait Time' for buffer to clear other wavelength data"
                # "Online"
                n157 = stacked-sequence {
                  frame #0 {
                    # "Read the online wavelength and continue adjusting the online DBR if outside the wavelength tolerance\nuntil it is within tolerance"
                    n158 = while {
                      i -> [w236]
                      stop <- w233 stop-if-true
                      # "Frame 2: Decrement DBR current if above tolerance\nFrame 3: Increment DBR current if below tolerance"
                      # "Frame 0: Read the current wavelength from the wavemeter\nFrame 1: Calculate the difference between desired and actual wavelength"
                      # "Continue reading and adjusting online DBR current until within locking tolerance"
                      n159 = local read "ILX Address On"() -> (w237:dbl)
                      n160 = stacked-sequence {
                        tunnel: w237 -> [_ _ _ w262 w281]
                        tunnel: w236 -> [w239 _ _ _ _]
                        tunnel: [_ _ w252 _ _] -> w234
                        frame #0 {
                          n161 = Equal To 0?(x=w239) -> (x = 0?=w238:bool)
                          n162 = case shown="True" w238 {
                            frame False {
                            }
                            frame True {
                              # "Set the TSOA switch to\namplify the ABSORBING\nwavelength"
                              n163 = Build Array(FALSE ("Boolean")) -> (w240:bool[])
                              n164 = call-poly <vilib>:"DAQmx Write.vi"("task/channels in"=refnum<k21> "BristolWM", "data"=w240) -> ()  [unwired: 11 in, 3 out]
                            }
                          }
                        }
                        frame #1 {
                          # "Reading the wavelength from the wavemeter"
                          n165 = flat-sequence {
                            tunnel: [w245] -> w244
                            tunnel: w244 -> [w248]
                            tunnel: [w247] -> w243
                            tunnel: w243 -> [w251]
                            frame #0 {
                              n166 = local read "Bristol In"() -> (w246:i32)
                              n167 = dll-call lib="C:/Users/H2ODial/Desktop/Shared Telescope WV DIAL Code/Libraries and VIs/CLDevIface.dll" fn="CLOpenUSBSerialDevice"("commPort"=w246) -> ("return type"=w245:i32)  [unwired: 4 in, 2 out]
                            }
                            frame #1 {
                              n168 = dll-call lib="C:/Users/H2ODial/Desktop/Shared Telescope WV DIAL Code/Libraries and VIs/CLDevIface.dll" fn="CLGetLambdaReading"("devHandle"=w248) -> ("return type"=→"Lambda On Read (nm)":dbl, "devHandle"=w247:i32)  [unwired: 3 in, 2 out]
                            }
                            frame #2 {
                              n169 = dll-call lib="C:/Users/H2ODial/Desktop/Shared Telescope WV DIAL Code/Libraries and VIs/CLDevIface.dll" fn="CLCloseDevice"("commPort"=w251) -> ("return type"=w250:i32)  [unwired: 4 in, 2 out]
                              n170 = local write "Bristol Out"(w250) -> ()
                            }
                          }
                        }
                        frame #2 {
                          # "If WL difference is within tolerance, stop looping, and illuminate 'Wavelength Lock Online' indicator"
                          # "Calculating the difference between the actual and desired online wavelength"
                          n171 = local read "Lambda On Read (nm)"() -> (w260:dbl)
                          n172 = local read "Online_Tol"() -> (w257:dbl)
                          n173 = Multiply(x=-1.0, y=w257) -> (x*y=w258:dbl)
                          n174 = Subtract(x=w260, y="Lambda On Set (nm)") -> (x-y=w253:dbl)
                          "WL_Difference" <- w253
                          n175 = Greater?(x=w253, y=w258) -> (0:w254:bool)
                          n176 = Less?(x=w253, y=w257) -> (x < y?=w255:bool)
                          n177 = And(x=w254, y=w255) -> (x .and. y?=w252:bool)
                          "Wavelength Lock Online" <- w252
                        }
                        frame #3 {
                          # "If the wavelength difference is greater that 0.0002 nm, decrement the \nDBR current by 0.01 mA"
                          n178 = local read "WL_Difference"() -> (w264:dbl)
                          n179 = Greater Or Equal?(x=w264, y="Online_Tol") -> (x >= y?=w263:bool)
                          n180 = case shown="True" w263 {
                            tunnel: w262 -> [_ w265]
                            frame False {
                              # "Wavelength difference is not greater than 0.0002 nm, do nothing"
                            }
                            frame True {
                              n181 = stacked-sequence {
                                tunnel: w265 -> [w266 w269]
                                frame #0 {
                                # "Specifying laser channel 1,\nwhich is the online channel"
                                n182 = Number To Decimal String(number=w266) -> (decimal integer string=w267:string)  [unwired: 1 in]
                                n183 = GPIB Write(0:w267, 1:"LAS:CHAN 2") -> ()  [unwired: 3 in, 2 out]
                                }
                                frame #1 {
                                # "issuing the command"
                                # "Generating a command string\nto decrement the current"
                                # "WL difference is greater than 0.0002 nm,\ndecrement the DBR current by 0.01 mA"
                                n184 = local read "Lambda On DBR Current"() -> (w276:dbl)
                                n185 = Subtract(x=w276, y=0.01) -> (x-y=w270:dbl)
                                n186 = local write "Lambda On DBR Current"(w270) -> ()
                                n187 = Format Into String(format string="%.4f" ("Format String"), w270) -> (resulting string=w273:string)  [unwired: 2 in, 1 out]
                                n188 = Concatenate Strings("LAS:LDI ", w273) -> (w272:string)
                                n189 = Number To Decimal String(number=w269) -> (decimal integer string=w271:string)  [unwired: 1 in]
                                n190 = GPIB Write(0:w271, 1:w272) -> ()  [unwired: 3 in, 2 out]
                                }
                              }
                            }
                          }
                        }
                        frame #4 {
                          # "If WL difference is < 0.0002 nm, increment the DBR current"
                          n191 = local read "Online_Tol"() -> (w279:dbl)
                          n192 = local read "WL_Difference"() -> (w283:dbl)
                          n193 = Multiply(x=-1.0, y=w279) -> (x*y=w278:dbl)
                          n194 = Less Or Equal?(x=w283, y=w278) -> (x <= y?=w282:bool)
                          n195 = case shown="True" w282 {
                            tunnel: w281 -> [_ w284]
                            frame False {
                              # "WL difference is no <= to -0.0002 nm, do nothing"
                            }
                            frame True {
                              n196 = stacked-sequence {
                                tunnel: w284 -> [w286 w288]
                                frame #0 {
                                # "Specifying laser channel 1,\nwhich is the online channel"
                                n197 = Number To Decimal String(number=w286) -> (decimal integer string=w285:string)  [unwired: 1 in]
                                n198 = GPIB Write(0:w285, 1:"LAS:CHAN 2") -> ()  [unwired: 3 in, 2 out]
                                }
                                frame #1 {
                                # "issuing the command"
                                # "Generating a command \nstring to increment the current"
                                # "WL difference is < -0.0002,\nincrement the DBR current by 0.01 mA"
                                n199 = local read "Lambda On DBR Current"() -> (w295:dbl)
                                n200 = Add(x=w295, y=0.01) -> (x+y=w290:dbl)
                                n201 = local write "Lambda On DBR Current"(w290) -> ()
                                n202 = Format Into String(format string="%.4f" ("Format String"), w290) -> (resulting string=w292:string)  [unwired: 2 in, 1 out]
                                n203 = Concatenate Strings("LAS:LDI ", w292) -> (w291:string)
                                n204 = Number To Decimal String(number=w288) -> (decimal integer string=w289:string)  [unwired: 1 in]
                                n205 = GPIB Write(0:w289, 1:w291) -> ()  [unwired: 3 in, 2 out]
                                }
                              }
                            }
                          }
                        }
                      }
                      n206 = Or(x=w234, y="Cancel online") -> (x .or. y?=w233:bool)
                    }
                  }
                  frame #1 {
                    # "Converting to pulse energy, assumes 5 percent pickoff"
                    # "Reading the Newport Power meter"
                    # "Reading the output power of the laser transmitter from the Newport power meter, once read, convert to corresponding pulse energy and plot"
                    n207 = local read "Newport Device Key"() -> (w301:string)
                    n208 = local read "NewportRef"() -> (w297:refnum<k24>)
                    n209 = disable-structure shown="Disabled" {
                      frame Disabled {
                        # "Plotting the online and offling pulse energies"
                        n210 = local read "Online Pulse Energy"() -> (w312:dbl)
                        n211 = local read "Offline Pulse Energy"() -> (w311:dbl)
                        n212 = Bundle("Online Pulse Energy"=w312, "Offline Pulse Energy"=w311) -> (→"Pulse Energy (Micro Joule)":T9)  [unwired: 1 in]
                      }
                      frame Enabled {
                      }
                    }
                    n213 = Number To Decimal String(number="SampleSize") -> (decimal integer string=w299:string)  [unwired: 1 in]
                    n214 = invoke class="PowerMeterCommands" method="PerformDAQ"(reference=w297, "deviceKey"=w301, "interval"="1", "sampleSize"=w299) -> ("PerformDAQ"=w302:dbl[])  [unwired: 2 in, 5 out]
                    n215 = call-poly <vilib>:"Mean.vi"("X"=w302) -> ("mean"=w300:dbl)  [unwired: 1 out]
                    n216 = Multiply(x=w300, y=1000.0) -> (x*y=w308:dbl)
                    n217 = Divide(x=w308, y=0.05) -> (x/y=w306:dbl)
                    n218 = Divide(x=w306, y=7.0) -> (x/y=→"Online Pulse Energy":dbl)
                  }
                  frame #2 {
                    # "Wait 'Scalar Wait Time' for the next available batch of scalar card data"
                    n219 = local read "AMCS_Profile"() -> (w313:i32)
                    n220 = disable-structure shown="Disabled" {
                      frame Disabled {
                        # "Waiting 'Scalar Wait Time'"
                        n221 = Wait (ms)(milliseconds to wait="Scalar Wait Time") -> ()  [unwired: 1 out]
                      }
                      frame Enabled {
                      }
                    }
                    n222 = while {
                      tunnel: [w320] -> w314
                      tunnel: [w316] -> _
                      tunnel: w313 -> [w316]
                      stop <- w318 stop-if-true
                      n223 = global read "AMCS_Data.vi" "AMCS_Profile"() -> (w320:i32)
                      n224 = Wait (ms)(milliseconds to wait=u32 10) -> ()  [unwired: 1 out]
                      n225 = Equal?(x=w320, y=w316) -> (x = y?=w319:bool)
                      n226 = case shown="False" w319 {
                        tunnel: [TRUE FALSE] -> w318
                        frame False {
                        }
                        frame True {
                        }
                      }
                    }
                    "AMCS_Profile" <- w314
                  }
                  frame #3 {
                    # "convert time per range bin to meters\nand calculate smoothed bins using\nsmoothing range"
                    # "Plotting online cross section and smoothed online data"
                    # "Calculate the bin by bin mean of the data"
                    # "Collect 'Integration Period (Seconds)' number\nof scalar data"
                    # "Reading, processing, and plotting the online data"
                    n227 = local read "Data Reads (number of loops)"() -> (w348:i32)
                    n228 = for {
                      N: w348 -> [_]
                      tunnel: [w369] -> w360 mode=indexing
                      tunnel: [w368] -> w323 mode=indexing
                      # "Scalar Data is retrieved from Global \nVariable that scaler.vi is writing to,"
                      n229 = global read "AMCS_Data.vi" "AMCS_Data"() -> (w372:u16[][])
                      n230 = disable-structure shown="Disabled" {
                        frame Disabled {
                          n231 = global read "Scalar_Data_3.vi" "Scalar Data 3"() -> ()  [unwired: 1 out]
                          n232 = global read "Scalar_Data.vi" "Scalar Data"() -> ()  [unwired: 1 out]
                        }
                        frame Enabled {
                        }
                      }
                      n233 = Index Array(array=w372, index (row) #1=0 ("index (row)"), index (row) #2=2 ("index (row)")) -> (element #1=w369:u16[], element #2=w368:u16[])  [unwired: 2 in]
                    }
                    n234 = Transpose 2D Array(2D array=w360) -> (transposed array=w364:u16[][])
                    n235 = Transpose 2D Array(2D array=w323) -> (transposed array=w346:u16[][])
                    n236 = for {
                      tunnel: w364 -> [w374] mode=indexing
                      tunnel: [w373] -> w365 mode=indexing
                      n237 = call-poly <vilib>:"Mean.vi"("X"=w374) -> ("mean"=w373:dbl)  [unwired: 1 out]
                    }
                    n238 = for {
                      tunnel: w346 -> [w367] mode=indexing
                      tunnel: [w366] -> w347 mode=indexing
                      n239 = call-poly <vilib>:"Mean.vi"("X"=w367) -> ("mean"=w366:dbl)  [unwired: 1 out]
                    }
                    n240 = local read "bins"() -> (w340:u32)
                    n241 = Array Subset(array=w365, index=1 ("dimension size"), length=w340) -> (w352:dbl[])
                    n242 = Array Subset(array=w347, index=1 ("dimension size"), length=w340) -> (w344:dbl[])
                    n243 = local read "background length"() -> (w330:i32)
                    n244 = local read "background start"() -> (w331:u32)
                    n245 = Array Size(array=w352) -> (size(s)=w349:i32)
                    n246 = Array Size(array=w344) -> (size(s)=w341:i32)
                    n247 = Initialize Array(1.0 ("element"), w349) -> (w351:dbl[])
                    n248 = Initialize Array(1.0 ("element"), w341) -> (w343:dbl[])
                    n249 = Multiply(x=w352, y=w351) -> (x*y=w353:dbl[])
                    "On-Line Bin Readings" <- w353
                    n250 = Multiply(x=w344, y=w343) -> (x*y=w334:dbl[])
                    "On-Line Bin Readings 2" <- w334
                    n251 = local read "Total DIAL Integration Time (Minutes)"() -> (w356:i32)
                    n252 = local read "Time Resolution Per Bin(ns)"() -> (w326:u32)
                    n253 = Array Subset(array=w353, index=w331, length=w330) -> (w362:dbl[])
                    n254 = Array Subset(array=w334, index=w331, length=w330) -> (w336:dbl[])
                    n255 = call-poly <vilib>:"Mean.vi"("X"=w362) -> ("mean"=w361:dbl)  [unwired: 1 out]
                    n256 = call-poly <vilib>:"Mean.vi"("X"=w336) -> ("mean"=w337:dbl)  [unwired: 1 out]
                    n257 = Divide(x=w356, y=w348) -> (x/y=w354:dbl)
                    n258 = local read "Index"() -> (w335:i32)
                    n259 = Subtract(x=w353, y=w361) -> (x-y=w358:dbl[])
                    n260 = Subtract(x=w334, y=w337) -> (x-y=w338:dbl[])
                    n261 = To Double Precision Float(number=w326) -> (double precision float=w327:dbl)
                    n262 = Multiply(x=w354, y=60.0) -> (x*y=w332:dbl)
                    n263 = Multiply(x=w327, y=0.15) -> (x*y=w329:dbl)
                    n264 = call "Ring Buffer Online Far.vi"("Index"=w335, "Profiles to Average"=w332, "Input Array"=w358) -> ("AvgArray"=w357:dbl[])  [unwired: 7 in, 1 out]
                    n265 = call "Ring Buffer Online Near.vi"("Index"=w335, "Profiles to Average"=w332, "Input Array"=w338) -> ("AvgArray"=w339:dbl[])  [unwired: 7 in, 1 out]
                    n266 = Divide(x="Smoothing Range", y=w329) -> (x/y=w324:dbl)
                    "Smoothed Bins" <- w324
                    n267 = call "Smooth Arrray.vi"("smooth size"=w324, "Raw Array"=w357) -> ("Smoothed Array"=→"On-Line  Smoothed":dbl[])  [unwired: 9 in]
                    n268 = call "Smooth Arrray.vi"("smooth size"=w324, "Raw Array"=w339) -> ("Smoothed Array"=→"On-Line Smoothed 2":dbl[])  [unwired: 9 in]
                    n269 = disable-structure shown="Disabled" {
                      frame Disabled {
                        n270 = script code="format long;\ncounts=sum(Online);\nif counts >=0.5e6\ntime=time;\nelse\ntime=time\nend"() -> ()  [unwired: 3 in, 2 out]
                      }
                      frame Enabled {
                      }
                    }
                  }
                  frame #4 {
                    # "Toggling the Agiltron switch to the offline DBR seed laser"
                    n271 = disable-structure shown="Disabled" {
                      frame Disabled {
                        n272 = flat-sequence {
                          frame #0 {
                            # "Second one"
                            # "Command the switch to switch to position 2\ncorresponding to the offline DBR"
                            # "Hex string command \ncorrespond to offline"
                            n273 = VISA Write(VISA resource name="Switch Comm Port", write buffer="\u0001\u0012\u0000\u0001") -> ()  [unwired: 1 in, 3 out]
                          }
                        }
                      }
                      frame Enabled {
                      }
                    }
                  }
                  frame #5 {
                    # "Save the recently collected online data if 'Save Data?' is true"
                    n274 = case shown="True" "Save Data?" {
                      frame False {
                        # "'Save Data?' is false, do nothing"
                      }
                      frame True {
                        # "'Save Data?' is true, save onfline data to the Data Disk"
                        # "Write only one copy of data at this time"
                        # "Retrieve Julian Date"
                        n275 = local read "Lambda On DBR Current"() -> (w402:dbl)
                        n276 = local read "Lambda On Read (nm)"() -> (w403:dbl)
                        n277 = local read "On-Line Bin Readings 2"() -> (w397:dbl[])
                        n278 = local read "Relative Humdity (%)"() -> (w398:dbl)
                        n279 = local read "On-Line Bin Readings"() -> (w405:dbl[])
                        n280 = local read "Online Pulse Energy"() -> (w401:dbl)
                        n281 = local read "Temperature (C)"() -> (w400:dbl)
                        n282 = local read "Pressure (mb)"() -> (w399:dbl)
                        n283 = call "Julian_Date_2.vi"() -> ("Julian Date"=w404:dbl)  [unwired: 11 in]
                        n284 = Build Array (concatenate)(w404, w403, w402, w401, w400, w399, w398, w405) -> (w392:dbl[])
                        n285 = Build Array (concatenate)(w404, w403, w402, w401, w400, w399, w398, w397) -> (w382:dbl[])
                        n286 = local write "DataOpen"(TRUE ("DataOpen")) -> ()
                        n287 = local read "NF_On_Ref"() -> (w380:refnum<file>)
                        n288 = local read "FF_On_Ref"() -> (w396:refnum<file>)
                        n289 = local read "NF_On_Ptr"() -> (w381:i64)
                        n290 = local read "FF_On_Ptr"() -> (w395:i64)
                        n291 = Set File Position(offset (in bytes) (0)=w395, refnum=w396) -> (refnum out=w393:refnum<file>, error out=w390:errorcluster)  [unwired: 2 in]
                        n292 = Set File Position(offset (in bytes) (0)=w381, refnum=w380) -> (refnum out=w386:refnum<file>, error out=w384:errorcluster)  [unwired: 2 in]
                        n293 = Write to Binary File(file (use dialog)=w386, data=w382, error in=w384, 5:FALSE ("prepend array or string size? (T)")) -> (refnum out=w385:refnum<file>, error out=w383:errorcluster)  [unwired: 2 in, 1 out]
                        n294 = Write to Binary File(file (use dialog)=w393, data=w392, error in=w390, 5:FALSE ("prepend array or string size? (T)")) -> (refnum out=w391:refnum<file>, error out=w389:errorcluster)  [unwired: 2 in, 1 out]
                        n295 = Get File Position(4:w383, 7:w385) -> (2:w379:i64)  [unwired: 2 out]
                        n296 = Get File Position(4:w389, 7:w391) -> (2:w388:i64)  [unwired: 2 out]
                        n297 = local write "NF_On_Ptr"(w379) -> ()
                        n298 = local write "FF_On_Ptr"(w388) -> ()
                      }
                    }
                  }
                }
              }
              frame #3 {
                # "Frame 3: Read offline data, calculate aerosol data, and plot offline and normalized relative backscatter\nFrame 4:\nFrame 5: Save the offline data and related information"
                # "Frame 0: Read the offline wavelength and lock if necessary, Switch to online DBR\nFrame 1: Read the output power from the Newport power meter\nFrame 2: Wait 'Scalar Wait Time' for buffers to clear of online contiminated data"
                # "offline"
                n299 = stacked-sequence {
                  frame #0 {
                    # "Every 60 data collection cycles, read the offline DBR wavelength, and if outside of wavelength tolerance, adjust DBR current until within tolerance"
                    n300 = local read "L_Count"() -> (w407:i32)
                    n301 = Quotient & Remainder(x=w407, y=60.0) -> (x-y*floor(x/y)=w408:dbl)  [unwired: 1 out]
                    n302 = Equal To 0?(x=w408) -> (x = 0?=w406:bool)
                    n303 = case shown="True" w406 {
                      frame False {
                      }
                      frame True {
                        n304 = while {
                          i -> [w413]
                          stop <- w411 stop-if-true
                          # "If WL difference is within tolerance, stop looping, and illuminate 'Wavelength Lock Offline' indicator"
                          # "Frame 2: Decrement DBR current if above tolerance\nFrame 3: Increment DBR current if below tolerance"
                          # "Frame 0: Read the current wavelength from the wavemeter\nFrame 1: Calculate the difference between desired and actual wavelength"
                          # "Continue reading and adjusting offline DBR current until within locking tolerance"
                          n305 = local read "ILX Address Off"() -> (w414:dbl)
                          n306 = stacked-sequence {
                            tunnel: w414 -> [_ _ _ w444 w460]
                            tunnel: w413 -> [w416 _ _ _ _]
                            tunnel: [_ _ w430 _ _] -> w410
                            frame #0 {
                              n307 = Equal To 0?(x=w416) -> (x = 0?=w415:bool)
                              n308 = case shown="True" w415 {
                                frame False {
                                }
                                frame True {
                                # "Set the TSOA switch to\namplify the non ABSORBING\nwavelength"
                                n309 = Build Array(TRUE ("Boolean")) -> (w418:bool[])
                                n310 = call-poly <vilib>:"DAQmx Write.vi"("task/channels in"=refnum<k21> "BristolWM", "data"=w418) -> ()  [unwired: 11 in, 3 out]
                                n311 = Wait (ms)(milliseconds to wait=u32 3200) -> ()  [unwired: 1 out]
                                }
                              }
                            }
                            frame #1 {
                              # "Reading the wavelength from the wavemeter"
                              n312 = flat-sequence {
                                tunnel: [w423] -> w422
                                tunnel: w422 -> [w426]
                                tunnel: [w425] -> w421
                                tunnel: w421 -> [w429]
                                frame #0 {
                                n313 = local read "Bristol In"() -> (w424:i32)
                                n314 = dll-call lib="C:/Users/H2ODial/Desktop/Shared Telescope WV DIAL Code/Libraries and VIs/CLDevIface.dll" fn="CLOpenUSBSerialDevice"("commPort"=w424) -> ("return type"=w423:i32)  [unwired: 4 in, 2 out]
                                }
                                frame #1 {
                                n315 = dll-call lib="C:/Users/H2ODial/Desktop/Shared Telescope WV DIAL Code/Libraries and VIs/CLDevIface.dll" fn="CLGetLambdaReading"("devHandle"=w426) -> ("return type"=→"Lambda Off Read (nm)":dbl, "devHandle"=w425:i32)  [unwired: 3 in, 2 out]
                                }
                                frame #2 {
                                n316 = dll-call lib="C:/Users/H2ODial/Desktop/Shared Telescope WV DIAL Code/Libraries and VIs/CLDevIface.dll" fn="CLCloseDevice"("commPort"=w429) -> ("return type"=w428:i32)  [unwired: 4 in, 2 out]
                                n317 = local write "Bristol Out"(w428) -> ()
                                }
                              }
                            }
                            frame #2 {
                              # "Calculating the difference between the actual and desired online wavelength"
                              n318 = local read "Offline_Tol"() -> (w432:dbl)
                              n319 = local read "Lambda Off Read (nm)"() -> (w438:dbl)
                              n320 = Multiply(x=-1.0, y=w432) -> (x*y=w431:dbl)
                              n321 = Subtract(x=w438, y="Lambda Off Set (nm)") -> (x-y=w434:dbl)
                              "WL Difference off" <- w434
                              n322 = Greater?(x=w434, y=w431) -> (0:w435:bool)
                              n323 = Less?(x=w434, y=w432) -> (x < y?=w436:bool)
                              n324 = And(x=w435, y=w436) -> (x .and. y?=w430:bool)
                              "Wavelength Lock Offline" <- w430
                              n325 = case shown="True" w430 {
                                frame False {
                                }
                                frame True {
                                # "Set the TSOA switch to\namplify the ABSORBING\nwavelength"
                                n326 = Build Array(FALSE ("Boolean")) -> (w440:bool[])
                                n327 = call-poly <vilib>:"DAQmx Write.vi"("task/channels in"=refnum<k21> "BristolWM", "data"=w440) -> ()  [unwired: 11 in, 3 out]
                                n328 = Wait (ms)(milliseconds to wait=u32 3200) -> ()  [unwired: 1 out]
                                }
                              }
                            }
                            frame #3 {
                              # "If the wavelength difference is greater that 0.0002 nm, decrement the \nDBR current by 0.01 mA"
                              n329 = local read "WL Difference off"() -> (w446:dbl)
                              n330 = Greater Or Equal?(x=w446, y="Offline_Tol") -> (x >= y?=w445:bool)
                              n331 = case shown="True" w445 {
                                tunnel: w444 -> [_ w447]
                                frame False {
                                # "Wavelength difference is not greater than 0.0002 nm, do nothing"
                                }
                                frame True {
                                n332 = stacked-sequence {
                                tunnel: w447 -> [w448 w451]
                                frame #0 {
                                # "Specifying laser channel 1,\nwhich is the online channel"
                                n333 = Number To Decimal String(number=w448) -> (decimal integer string=w449:string)  [unwired: 1 in]
                                n334 = GPIB Write(0:w449, 1:"LAS:CHAN 2") -> ()  [unwired: 3 in, 2 out]
                                }
                                frame #1 {
                                # "issuing the command"
                                # "Generating a command string\nto decrement the current"
                                # "WL difference is greater than 0.0002 nm,\ndecrement the DBR current by 0.01 mA"
                                n335 = local read "Lambda Off DBR Current"() -> (w458:dbl)
                                n336 = Subtract(x=w458, y=0.01) -> (x-y=w452:dbl)
                                n337 = local write "Lambda Off DBR Current"(w452) -> ()
                                n338 = Format Into String(format string="%.4f" ("Format String"), w452) -> (resulting string=w455:string)  [unwired: 2 in, 1 out]
                                n339 = Concatenate Strings("LAS:LDI ", w455) -> (w454:string)
                                n340 = Number To Decimal String(number=w451) -> (decimal integer string=w453:string)  [unwired: 1 in]
                                n341 = GPIB Write(0:w453, 1:w454) -> ()  [unwired: 3 in, 2 out]
                                }
                                }
                                }
                              }
                            }
                            frame #4 {
                              # "If WL difference is < 0.0002 nm, increment the DBR current"
                              n342 = local read "WL Difference off"() -> (w463:dbl)
                              n343 = Less Or Equal?(x=w463, y=-0.0001) -> (x <= y?=w461:bool)
                              n344 = case shown="True" w461 {
                                tunnel: w460 -> [_ w464]
                                frame False {
                                # "WL difference is no <= to -0.0002 nm, do nothing"
                                }
                                frame True {
                                n345 = stacked-sequence {
                                tunnel: w464 -> [w466 w468]
                                frame #0 {
                                # "Specifying laser channel 1,\nwhich is the online channel"
                                n346 = Number To Decimal String(number=w466) -> (decimal integer string=w465:string)  [unwired: 1 in]
                                n347 = GPIB Write(0:w465, 1:"LAS:CHAN 2") -> ()  [unwired: 3 in, 2 out]
                                }
                                frame #1 {
                                # "issuing the command"
                                # "Generating a command \nstring to increment the current"
                                # "WL difference is < -0.0002,\nincrement the DBR current by 0.01 mA"
                                n348 = local read "Lambda Off DBR Current"() -> (w475:dbl)
                                n349 = Add(x=w475, y=0.01) -> (x+y=w470:dbl)
                                n350 = local write "Lambda Off DBR Current"(w470) -> ()
                                n351 = Format Into String(format string="%.4f" ("Format String"), w470) -> (resulting string=w472:string)  [unwired: 2 in, 1 out]
                                n352 = Concatenate Strings("LAS:LDI ", w472) -> (w471:string)
                                n353 = Number To Decimal String(number=w468) -> (decimal integer string=w469:string)  [unwired: 1 in]
                                n354 = GPIB Write(0:w469, 1:w471) -> ()  [unwired: 3 in, 2 out]
                                }
                                }
                                }
                              }
                            }
                          }
                          n355 = Or(x=w410, y="Cancel Offline") -> (x .or. y?=w411:bool)
                        }
                      }
                    }
                  }
                  frame #1 {
                    # "Reading the power meter"
                    # "Updating the pulse energy plot"
                    # "Converting to pulse energy"
                    # "Reading the offline output power, converting to pulse energy,  and updating the Pulse energy plot"
                    n356 = local read "SampleSize"() -> (w479:i32)
                    n357 = local read "Newport Device Key"() -> (w480:string)
                    n358 = local read "Online Pulse Energy"() -> (w486:dbl)
                    n359 = local read "Offline Pulse Energy"() -> (w485:dbl)
                    n360 = local read "NewportRef"() -> (w477:refnum<k24>)
                    n361 = Number To Decimal String(number=w479) -> (decimal integer string=w481:string)  [unwired: 1 in]
                    n362 = invoke class="PowerMeterCommands" method="PerformDAQ"(reference=w477, "deviceKey"=w480, "interval"="1", "sampleSize"=w481) -> ("PerformDAQ"=w482:dbl[])  [unwired: 2 in, 5 out]
                    n363 = Bundle("Online Pulse Energy"=w486, "Offline Pulse Energy"=w485) -> (w484:T9)  [unwired: 1 in]
                    n364 = local write "Pulse Energy (Micro Joule)"(w484) -> ()
                    n365 = call-poly <vilib>:"Mean.vi"("X"=w482) -> ("mean"=w478:dbl)  [unwired: 1 out]
                    n366 = Multiply(x=w478, y=1000.0) -> (x*y=w491:dbl)
                    n367 = Divide(x=w491, y=0.05) -> (x/y=w489:dbl)
                    n368 = Divide(x=w489, y=7.0) -> (x/y=→"Offline Pulse Energy":dbl)
                  }
                  frame #2 {
                    # "Wait 'Scalar Wait Time' for buffers to clear of online contiminated offline data"
                    n369 = disable-structure shown="Disabled" {
                      frame Disabled {
                        # "Wait 'Scalar Wait Time'"
                        n370 = local read "Scalar Wait Time"() -> (w493:u32)
                        n371 = Wait (ms)(milliseconds to wait=w493) -> ()  [unwired: 1 out]
                      }
                      frame Enabled {
                      }
                    }
                  }
                  frame #3 {
                    w527 = 1 ("dimension size")
                    w531 = 1
                    # "Read in latest scalar card data from \n'Scalar Data' global variable that \nscaler.vi is writing to, then wait 1 sec\nfor next batch of data"
                    # "Plotting the normalized relative \nbackscatter"
                    # "Calculating the normalized relative backscatter"
                    # "Calculating/Plotting smoothed data,\ncross sections etc."
                    # "Pick off data with\nout header"
                    # "Calculate mean bin by bin mean"
                    # "Reading in 'Integration Period (Seconds)' of data"
                    # "Read the offline data from the scalar card, perform smoothing, calculate normalized relative backscatter, and plot"
                    # "File path in MATLAB script is of old dial is:\nF:\\Micropulse DIAL\\Micropulse DIAL Matlab\\\nFinal Overlap Function.mat')];"
                    # "Collects Data From Card,\nSends It To The Chart,\nAnd Saves A Copy As A\nFile If Option Selected On\nFront Panel"
                    n372 = for {
                      N: "Data Reads (number of loops)" -> [_]
                      tunnel: [w563] -> w495 mode=indexing
                      tunnel: [w562] -> w494 mode=indexing
                      n373 = global read "AMCS_Data.vi" "AMCS_Data"() -> (w564:u16[][])
                      n374 = disable-structure shown="Disabled" {
                        frame Disabled {
                          n375 = global read "Scalar_Data_4.vi" "Scalar Data 4"() -> ()  [unwired: 1 out]
                          n376 = global read "Scalar_Data_2.vi" "Scalar Data 2"() -> ()  [unwired: 1 out]
                        }
                        frame Enabled {
                        }
                      }
                      n377 = Index Array(array=w564, index (row) #1=1 ("index (row)"), index (row) #2=3 ("index (row)")) -> (element #1=w563:u16[], element #2=w562:u16[])  [unwired: 2 in]
                    }
                    n378 = local read "Total DIAL Integration Time (Minutes)"() -> (w552:i32)
                    n379 = Divide(x=w552, y="Data Reads (number of loops)") -> (x/y=w550:dbl)
                    n380 = local read "Total Aerosol Integration Time (Minutes)"() -> (w554:dbl)
                    n381 = local read "background length"() -> (w499:i32)
                    n382 = Multiply(x=w550, y=60.0) -> (x*y=w537:dbl)
                    n383 = local read "background start"() -> (w500:u32)
                    n384 = Transpose 2D Array(2D array=w495) -> (transposed array=w560:u16[][])
                    n385 = Transpose 2D Array(2D array=w494) -> (transposed array=w543:u16[][])
                    n386 = Divide(x=w554, y="Data Reads (number of loops)") -> (x/y=w555:dbl)
                    n387 = for {
                      tunnel: w560 -> [w570] mode=indexing
                      tunnel: [w569] -> w561 mode=indexing
                      tunnel: w543 -> [w568] mode=indexing
                      tunnel: [w567] -> _ mode=indexing
                      tunnel: [w567] -> w540 mode=indexing
                      n388 = call-poly <vilib>:"Mean.vi"("X"=w570) -> ("mean"=w569:dbl)  [unwired: 1 out]
                      n389 = call-poly <vilib>:"Mean.vi"("X"=w568) -> ("mean"=w567:dbl)  [unwired: 1 out]
                    }
                    n390 = local read "bins"() -> (w528:u32)
                    n391 = Multiply(x=w555, y=60.0) -> (x*y=w518:dbl)
                    n392 = Array Subset(array=w540, index=w527, length=w528) -> (w541:dbl[])
                    "Off-Line Bin Readings 2" <- w541
                    n393 = Array Subset(array=w561, index=w527, length=w528) -> (w539:dbl[])
                    "Off-Line  Bin Readings" <- w539
                    n394 = Array Subset(array=w541, index=w500, length=w499) -> (w542:dbl[])
                    n395 = Array Subset(array=w539, index=w500, length=w499) -> (w559:dbl[])
                    n396 = local read "Smoothed Bins"() -> (w496:dbl)
                    n397 = call-poly <vilib>:"Mean.vi"("X"=w542) -> ("mean"=w506:dbl)  [unwired: 1 out]
                    n398 = call-poly <vilib>:"Mean.vi"("X"=w559) -> ("mean"=w507:dbl)  [unwired: 1 out]
                    n399 = local read "Index"() -> (w517:i32)
                    n400 = Subtract(x=w541, y=w506) -> (x-y=w519:dbl[])
                    n401 = Subtract(x=w539, y=w507) -> (x-y=w535:dbl[])
                    n402 = call "Ring Buffer Offline Far.vi"("Index"=w517, "Profiles to Average"=w537, "Input Array"=w535) -> ("AvgArray"=w557:dbl[], "RingBufferOut"=→"RingBuffer offline far":dbl[][])  [unwired: 7 in]
                    n403 = call "Ring Buffer Aerosol Far.vi"("Index"=w517, "Profiles to Average"=w518, "Input Array"=w535) -> ("AvgArray"=w553:dbl[], "RingBufferOut"=→"RingBuffer aerosol far":dbl[][])  [unwired: 7 in]
                    n404 = call "Ring Buffer Offline Near.vi"("Index"=w517, "Profiles to Average"=w537, "Input Array"=w519) -> ("AvgArray"=w538:dbl[], "RingBufferOut"=→"RingBuffer offline near":dbl[][])  [unwired: 7 in]
                    n405 = call "Ring Buffer Aerosol Near.vi"("Index"=w517, "Profiles to Average"=w518, "Input Array"=w519) -> ("AvgArray"=w515:dbl[], "RingBufferOut"=→"RingBuffer aerosol near":dbl[][])  [unwired: 7 in]
                    n406 = Reshape Array(w535, w527, w528) -> (→"raw counts":dbl[][])
                    n407 = Reshape Array(w519, w527, w528) -> (→"raw counts near":dbl[][])
                    n408 = call "Smooth Arrray.vi"("smooth size"=w496, "Raw Array"=w557) -> ("Smoothed Array"=→"Off-Line Smoothed":dbl[])  [unwired: 9 in]
                    n409 = call "Smooth Arrray.vi"("smooth size"=w496, "Raw Array"=w553) -> ("Smoothed Array"=w526:dbl[])  [unwired: 9 in]
                    "Aerosol Smoothed" <- w526
                    n410 = call "Smooth Arrray.vi"("smooth size"=w496, "Raw Array"=w538) -> ("Smoothed Array"=→"Off-Line Smoothed 2":dbl[])  [unwired: 9 in]
                    n411 = call "Smooth Arrray.vi"("smooth size"=w496, "Raw Array"=w515) -> ("Smoothed Array"=w498:dbl[])  [unwired: 9 in]
                    "Aerosol Smoothed 2" <- w498
                    n412 = local read "Number of Accumulates"() -> (w502:u32)
                    n413 = local read "Temperature (C)"() -> (w549:dbl)
                    n414 = local read "Pressure (mb)"() -> (w548:dbl)
                    n415 = script code="%accum_num=10000;     % scaler card setting number of accumulations\nt_bin = 500e-9                 % scaler card setting time per bin\n%t_d = 37.3e-9;                % APD dead time from spec sheet\n\n% conversion from accumulated counts to count rate  (c/s)\nc_convert = 1./t_bin./accum_num;\nCR_far = p_raw_far.*c_convert;\nCR_near = p_raw_near.*c_convert;\nCR_total_far = (p_raw_far+b_far).*c_convert;\nCR_total_near = (p_raw_near+b_near).*c_convert;\nb_CR_far =b_far.*c_convert;\nb_CR_near =b_near.*c_convert;\n\n% create a range array\nsize_p =  size(p_raw_far,2);\nr = (75:75:size_p*75)./1e3; \n    \n%APD correction factor\n D_far = 1./(1-(t_d*CR_total_far));\n D_near = 1./(1-(t_d*CR_total_near));\n\n %Calculating normalize relative backscatter profile\n nrb_far = CR_far.*D_far.*r.^2./E.*1e-6;\n nrb_near = CR_near.*D_near.*r.^2./E.*1e-6;"("E"=6.0 ("Real"), "temp"=w549, "press"=w548, "p_raw_far"=w526, "b_far"=w507, "b_near"=w506, "p_raw_near"=w498, "accum_num"=w502, "t_d"="dead time") -> ("nrb_far"=w521:cdb[], "D_far"=w512:dbl[], "nrb_near"=w520:cdb[], "D_near"=w511:dbl[], "b_CR_far"=w504:dbl, "b_CR_near"=w503:dbl)  [unwired: 1 in, 1 out]
                    n416 = local read "bins"() -> (w530:u32)
                    n417 = local read "Altitude Array (km)"() -> (w523:dbl[])
                    n418 = Bundle(w504, w503) -> (→"?":cluster{dbl, dbl})  [unwired: 1 in]
                    n419 = Build Array(w521, w520) -> (w525:cdb[][])
                    n420 = Build Array(w512, w511) -> (w510:dbl[][])
                    n421 = Reshape Array(w520, w531, w530) -> (→"NRB 2":cdb[][])
                    n422 = Reshape Array(w521, w531, w530) -> (→"NRB":cdb[][])
                    n423 = Build Array(w523, w523) -> (w522:dbl[][])
                    n424 = call "Convert to Dynamic Data7"("2D Array"=w510) -> ("Dynamic Data Type"=w509:dynamicdata)  [unwired: 3 in]
                    n425 = call "Convert to Dynamic Data3"("2D Array"=w525) -> ("Dynamic Data Type"=w524:dynamicdata)  [unwired: 3 in]
                    n426 = call "Convert to Dynamic Data4"("2D Array"=w522) -> ("Dynamic Data Type"=w513:dynamicdata)  [unwired: 3 in]
                    n427 = call "Build XY Graph2"("Y Input"=w513, "X Input"=w524) -> ("XY Graph"=→"NRB plot":cluster{"Y":dbl[], "Y":dbl[]}[])  [unwired: 3 in, 6 out]
                    n428 = call "Build XY Graph4"("Y Input"=w513, "X Input"=w509) -> ("XY Graph"=→"Correction":cluster{"Y":dbl[], "Y":dbl[]}[])  [unwired: 3 in, 6 out]
                  }
                  frame #4 {
                    # "REPLACE WITH NEW AGILTRON TASK!"
                    # "Toggle Agiltron switch to online DBR"
                    n429 = disable-structure shown="Disabled" {
                      frame Disabled {
                        # "ABSORBING"
                        n430 = flat-sequence {
                          frame #0 {
                            # "Third one"
                            # "Command the switch to switch to position 1\ncorresponding to the online DBR"
                            # "Hex string command \ncorrespond to online"
                            n431 = local read "Switch Comm Port"() -> (w574:refnum<visa-resource-name>)
                            n432 = VISA Write(VISA resource name=w574, write buffer="\u0001\u0012\u0000\u0002") -> ()  [unwired: 1 in, 3 out]
                          }
                        }
                        n433 = Build Array(FALSE ("Boolean")) -> (w573:bool[])
                        n434 = call-poly <vilib>:"DAQmx Write.vi"("task/channels in"=refnum<k21> "AgiltronSwitch", "data"=w573) -> ()  [unwired: 11 in, 3 out]
                      }
                      frame Enabled {
                      }
                    }
                  }
                  frame #5 {
                    # "If 'Save Data?' is true, save all relavant offline info"
                    n435 = local read "Save Data?"() -> (w576:bool)
                    n436 = case shown="True" w576 {
                      frame False {
                        # "'Save Data?' is false, do nothing"
                      }
                      frame True {
                        # "Write only one data file at this time"
                        # "Retrive Julian Date"
                        # "'Save Data?' is true, save offline data to the Data Disk"
                        n437 = local read "Lambda Off DBR Current"() -> (w598:dbl)
                        n438 = local read "Off-Line Bin Readings 2"() -> (w595:dbl[])
                        n439 = local read "Lambda Off Read (nm)"() -> (w597:dbl)
                        n440 = local read "Off-Line  Bin Readings"() -> (w603:dbl[])
                        n441 = local read "Relative Humdity (%)"() -> (w602:dbl)
                        n442 = local read "Offline Pulse Energy"() -> (w599:dbl)
                        n443 = local read "Temperature (C)"() -> (w600:dbl)
                        n444 = local read "Pressure (mb)"() -> (w601:dbl)
                        n445 = call "Julian_Date_2.vi"() -> ("Julian Date"=w596:dbl)  [unwired: 11 in]
                        n446 = Build Array (concatenate)(w596, w597, w598, w599, w600, w601, w602, w603) -> (w581:dbl[])
                        n447 = Build Array (concatenate)(w596, w597, w598, w599, w600, w601, w602, w595) -> (w578:dbl[])
                        n448 = local read "FF_Off_Ref"() -> (w583:refnum<file>)
                        n449 = local read "NF_Off_Ref"() -> (w580:refnum<file>)
                        n450 = local read "FF_Off_Ptr"() -> (w582:i64)
                        n451 = local read "NF_Off_Ptr"() -> (w579:i64)
                        n452 = Set File Position(offset (in bytes) (0)=w582, refnum=w583) -> (refnum out=w594:refnum<file>, error out=w592:errorcluster)  [unwired: 2 in]
                        n453 = Set File Position(offset (in bytes) (0)=w579, refnum=w580) -> (refnum out=w590:refnum<file>, error out=w588:errorcluster)  [unwired: 2 in]
                        n454 = Write to Binary File(file (use dialog)=w594, data=w581, error in=w592, 5:FALSE ("prepend array or string size? (T)")) -> (refnum out=w593:refnum<file>, error out=w591:errorcluster)  [unwired: 2 in, 1 out]
                        n455 = Write to Binary File(file (use dialog)=w590, data=w578, error in=w588, 5:FALSE ("prepend array or string size? (T)")) -> (refnum out=w589:refnum<file>, error out=w587:errorcluster)  [unwired: 2 in, 1 out]
                        n456 = Get File Position(4:w591, 7:w593) -> (2:w584:i64)  [unwired: 2 out]
                        n457 = Get File Position(4:w587, 7:w589) -> (2:w577:i64)  [unwired: 2 out]
                        n458 = local write "FF_Off_Ptr"(w584) -> ()
                        n459 = local write "NF_Off_Ptr"(w577) -> ()
                      }
                    }
                  }
                }
              }
              frame #4 {
                n460 = First Call?() -> (First Call?: T/F=w606:bool)
                n461 = Or(x="calculate absorption cross sections", y=w606) -> (x .or. y?=w604:bool)
                n462 = case shown="True" w604 {
                  frame False {
                  }
                  frame True {
                    # "calculate absorption cross sections from HITRAN data base"
                    n463 = local read "Off-Line Smoothed"() -> (w607:dbl[])
                    n464 = local read "Lambda On Read (nm)"() -> (w610:dbl)
                    n465 = local read "Lambda Off Set (nm)"() -> (w613:dbl)
                    n466 = local read "Temperature (C)"() -> (w611:dbl)
                    n467 = local read "Pressure (mb)"() -> (w612:dbl)
                    n468 = script code="%Importing HITRAN data\n%hitran = dlmread('C:\\Users\\H2ODial\\Desktop\\Shared Telescope WV DIAL Code\\Libraries and VIs\\824nm_841nm_H2O.csv', ',',[0 1 352 7]);\nhitran = dlmread('C:\\Users\\H2ODial\\Desktop\\Shared Telescope WV DIAL Code\\Libraries and VIs\\824nm_841nm_H2O_Spectral_Calc.csv', ',',[1 1 1209 7]);\n\n%Range vector in meters\nrange = ([75:75:size(Online,2)*75]);\n\nif lambda< 828\nlambda=828.195;\nelse\nlambda=lambda;\nend;\n\n%%\n\n%Voigt profile calculation\nWNmin = 12070.0;\nWNmax = 12076.0;\n\n%Find lines from WNmin to WNmax to calculate voigt profile\nline_indices = find(hitran(1:size(hitran,1),1)>WNmin & hitran(1:size(hitran,1),1)<WNmax);\n\nline = (hitran(line_indices, 1:size(hitran,2)));\n\n%Calculate temperature and pressure profile\nT0 = 273+15.6;\nT0 = 273+T0_C;\n\nT = T0-0.005545.*range; \n\nP0  = 1.0;\nP0  = P0_mb/1000*0.986; %pressure in mb converted to atm\n\nP = P0.*(T0./T).^-5.21986;\n\n%linewidth temperature dependence factor\nalpha = line(:,7);        \n\n%initial Lorentz linewidth from HiTRAN [cm^-1]\ngammal0 = line(:,4);     \n\n%ground state transition energy [cm^-1]\nE = line(:,6);           \n\n%initial linestrength from HiTRAN [cm^-1/(mol*cm^-2)]\nS0 = line(:,2);      \n\n%absorption line center wavenumber from HiTRAN [cm^-1]\nnu0_0 = line(:,1);    \n\nnu_on = (1/(lambda)*1e7);\n\nnu_off = (1/(lambda_off)*1e7);\n\n\nfor i = 1:size(Online,2);\n\n    %Pressure shift\n    nu0 = nu0_0-.0428.*P(i);\n    \n    %Calculate Lorentz lineweidth at temperature T [cm^-1]\n    gammal = gammal0.*(P(i)./P0).*((T0./T(i)).^alpha);\n    \n    %Calculate Doppler linewidth at temperature T [cm^-1]\n    gammad = (nu0).*((2.0.*1.38E-23.*T(i).*log(2.0))./(0.018.*3.0E8.*3.0E8./6.022E23)).^(0.5);\n    \n    y = (gammal./gammad).*((log(2.0)).^(0.5));\n    \n    x_on = ((nu_on-nu0)./gammad).*(log(2.0)).^(0.5);\n    \n    x_off = ((nu_off-nu0)./gammad).*(log(2.0)).^(0.5);\n    \n    %setting up Voigt convolution\n    stepsize = 1;\n    \n    t = [-200:1:199].*stepsize;\n    \n    t = repmat(t',1,length(x_on))';\n    \n    x_on = repmat(x_on,1,length(t));\n    \n    x_off = repmat(x_off,1,length(t));\n    \n    y = repmat(y,1,length(t));\n    \n    f_on = (exp(-t.^2.0))./(y.^2.0+(x_on-t).^2.0);\n    \n    f_off = (exp(-t.^2.0))./(y.^2.0+(x_off-t).^2.0);\n    \n    %Set the integration sum to zero to start\n    integral_on = 0.0;\n    \n    integral_off = 0.0;\n    \n    %Voigt integration\n    z_on = trapz(t(1,:),f_on,2);\n    \n    z_off =  trapz(t(1,:),f_off,2);\n    \n    integral_on = z_on;\n    \n    integral_off = z_off;\n    \n    %Calculate linestrength at temperature T\n    S = S0.*((T0./T(i)).^(1.5)).*exp(1.439.*E.*((1./T0)-(1./T(i))));\n    \n    %Calculate Doppler line-center cross section [cm^2]\n    K = (S./gammad).*(((log(2.0))./pi).^(0.5));\n    \n    %Calculate the Voigt profile\n    V_on = (y(1)/pi).*integral_on;\n    \n    V_off = (y(1)./pi).*integral_off;\n    \n    %Calculate the Voigt profile absorption cross section [cm^2]\n    sigmav_on = K.*V_on;\n    \n    sigmav_off = K.*V_off;\n    \n    %Sum contributions from all of the surrounding lines\n    sigma_on_total(i) = sum(sigmav_on);\n    \n    sigma_off_total(i) = sum(sigmav_off);\n    \nend;"("lambda"=w610, "lambda_off"=w613, "P0_mb"=w612, "T0_C"=w611, "Online"=w607) -> ("sigma_on_total"=→"sigma_on_total":dbl[], "sigma_off_total"=→"sigma_off_total":dbl[])  [unwired: 1 in, 1 out]
                  }
                }
              }
              frame #5 {
                w624 = 1
                # "normalization factor\nfrom 300 to 450m"
                # "OPTICAL DEPTH PLOT"
                # "new rainbow color bar display"
                # "Data Processing Far Channel"
                # "new rainbow color bar display"
                # "Calculating the range resolved water vapor number density and plotting"
                n469 = local read "sigma_off_total"() -> (w647:dbl[])
                n470 = local read "sigma_on_total"() -> (w644:dbl[])
                n471 = local read "On-Line  Smoothed"() -> (w622:dbl[])
                n472 = local read "Off-Line Smoothed"() -> (w621:dbl[])
                n473 = local read "Off-Line Smoothed 2"() -> (w645:dbl[])
                n474 = local read "On-Line Smoothed 2"() -> (w646:dbl[])
                n475 = script code="%Time averaging in seconds.  600 Seconds =10 minutes\ntemporal_average = 600;\n\n%Spatial averaging in bins.  2 bins = 150 meters\nspatial_average = 2;\n\n%Creating r and r+deltar vectors..this can also be acsomplished using the\n%diff command\np_oni = Online(:,1:size(Online,2)-1);\n\np_onii = Online(:,2:size(Online,2));\n\np_offi = Offline(:,1:size(Offline,2)-1);\n\np_offii = Offline(:,2:size(Offline,2));\n\nInside = (p_oni.*p_offii)./(p_onii.*p_offi);\n\ndel_cross = 1./(2.*(sigma_on_total(1:size(Online,2)-1)-sigma_off_total(1:size(Offline,2)-1)).*75*100);\n\ndel_cross(isinf(del_cross)) = 0;\n\n%Calculating Number density\nN = del_cross.*log(Inside);\n\n%Spatial smoothing of the profiles\nfilter1 = ones(1,2)./2;\n\nN_1 = N;\n\nN_1_avg = filter2(filter1,N_1);\n\nfilter1 = ones(1,10)./10;\n\nN_2 = N;\n\nN_2_avg = filter2(filter1,N_2);\n\nN_new = zeros(size(N,1),size(N,2));\n \n%Using different averaging windows for different altitudes \nN_avg=[N_1_avg(:,1:40)';N_2_avg(:,41:size(N,2))']';\n\n\nw = N_avg.*1e6.*18.015./6.022e23"("Online"=w646, "Offline"=w645, "sigma_on_total"=w644, "sigma_off_total"=w647) -> ("N_avg"=w648:cdb[], "w"=w657:cdb[])  [unwired: 1 in, 1 out]
                n476 = script code="%Time averaging in seconds.  600 Seconds = 10 minutes\ntemporal_average = 600;\n\n%Spatial averaging in bins.  2 bins = 150 meters\nspatial_average = 2;\n\n%Creating r and r+deltar vectors..this can also be acsomplished using the\n%diff command\np_oni = Online(:,1:size(Online,2)-1);\n\np_onii = Online(:,2:size(Online,2));\n\np_offi = Offline(:,1:size(Offline,2)-1);\n\np_offii = Offline(:,2:size(Offline,2));\n\nInside = (p_oni.*p_offii)./(p_onii.*p_offi);\n\ndel_cross = 1./(2.*(sigma_on_total(1:size(Online,2)-1)-sigma_off_total(1:size(Offline,2)-1)).*75*100);\n\ndel_cross(isinf(del_cross)) = 0;\n\n%Calculating Number density\nN = del_cross.*log(Inside);\n\n%Spatial smoothing of the profiles\nfilter1 = ones(1,2)./2;\n\nN_1 = N;\n\nN_1_avg = filter2(filter1,N_1);\n\nfilter1 = ones(1,10)./10;\n\nN_2 = N;\n\nN_2_avg = filter2(filter1,N_2);\n\nN_new = zeros(size(N,1),size(N,2));\n \n%Using different averaging windows for different altitudes \nN_avg=[N_1_avg(:,1:40)';N_2_avg(:,41:size(N,2))']';\n\n \nw = N_avg.*1e6.*18.015./6.022e23"("Online"=w622, "Offline"=w621, "sigma_on_total"=w644, "sigma_off_total"=w647) -> ("N_avg"=w653:cdb[], "w"=w654:cdb[])  [unwired: 1 in, 1 out]
                n477 = local read "Time Resolution Per Bin(ns)"() -> (w623:u32)
                n478 = local read "bins"() -> (w649:u32)
                n479 = local read "Altitude Array (km)"() -> (w619:dbl[])
                n480 = Build Array(w654, w657) -> (w660:cdb[][])
                n481 = To Double Precision Float(number=w623) -> (double precision float=w642:dbl)
                n482 = Reshape Array(w653, w624, w649) -> (w664:cdb[][])
                n483 = Reshape Array(w648, w624, w649) -> (w651:cdb[][])
                n484 = Multiply(x=0.15, y=w642) -> (x*y=w640:dbl)
                n485 = Build Array(w653, w648) -> (w658:cdb[][])
                n486 = Divide(x=300.0, y=w640) -> (x/y=w637:dbl)
                n487 = Divide(x=450.0, y=w640) -> (x/y=w636:dbl)
                n488 = Build Array(w619, w619) -> (w643:dbl[][])
                n489 = call "Convert to Dynamic Data5"("2D Array"=w660) -> ("Dynamic Data Type"=w659:dynamicdata)  [unwired: 3 in]
                n490 = call "Convert to Dynamic Data2"("2D Array"=w658) -> ("Dynamic Data Type"=w655:dynamicdata)  [unwired: 3 in]
                n491 = Divide(x=w664, y=1e+17) -> (x/y=→"Water Vapor Number Density":cdb[][])
                n492 = Divide(x=w651, y=1e+17) -> (x/y=→"Water Vapor Number Density 2":cdb[][])
                n493 = call "Convert to Dynamic Data6"("Array"=w619) -> ("Dynamic Data Type"=w620:dynamicdata)  [unwired: 3 in]
                n494 = To Long Integer(number=w637) -> (32bit integer=w635:i32)
                n495 = To Long Integer(number=w636) -> (32bit integer=w634:i32)
                n496 = call "Convert to Dynamic Data"("2D Array"=w643) -> ("Dynamic Data Type"=w656:dynamicdata)  [unwired: 3 in]
                n497 = call "Convert to Dynamic Data8"("2D Array"=w643) -> ("Dynamic Data Type"=w661:dynamicdata)  [unwired: 3 in]
                n498 = Decrement(x=w635) -> (x-1=w632:i32)
                n499 = Decrement(x=w634) -> (x-1=w633:i32)
                n500 = call "Build XY Graph"("Y Input"=w656, "X Input"=w655) -> ("XY Graph"=→"Water Vapor Number Density  2":cluster{"Y":dbl[], "Y":dbl[]}[])  [unwired: 3 in, 6 out]
                n501 = call "Build XY Graph3"("Y Input"=w661, "X Input"=w659) -> ("XY Graph"=→"Absolute Humidity":cluster{"Y":dbl[], "Y":dbl[]}[])  [unwired: 3 in, 6 out]
                n502 = Array Subset(array=w622, index=w632, length=w633) -> (w631:dbl[])
                n503 = Array Subset(array=w621, index=w632, length=w633) -> (w630:dbl[])
                n504 = call-poly <vilib>:"Mean.vi"("X"=w631) -> ("mean"=w629:dbl)  [unwired: 1 out]
                n505 = call-poly <vilib>:"Mean.vi"("X"=w630) -> ("mean"=w628:dbl)  [unwired: 1 out]
                n506 = Divide(x=w629, y=w628) -> (x/y=w627:dbl)
                n507 = Multiply(x=w621, y=w627) -> (x*y=w626:dbl[])
                n508 = Divide(x=w622, y=w626) -> (x/y=w625:dbl[])
                n509 = Natural Logarithm(1:w625) -> (0:w616:dbl[])
                n510 = Multiply(x=-1.0, y=w616) -> (x*y=w615:dbl[])
                n511 = call "Convert to Dynamic Data9"("Array"=w615) -> ("Dynamic Data Type"=w618:dynamicdata)  [unwired: 3 in]
                n512 = call "Build OD Plot"("Y Input"=w620, "X Input"=w618) -> ("XY Graph"=→"Optical Depth":cluster{"Y":dbl[], "Y":dbl[]}[])  [unwired: 3 in, 6 out]
              }
            }
          }
        }
        "L_Count" <- w126
      }
    }
  }
  n513 = case shown="True" w3 {
    frame False {
    }
    frame True {
      # "close data files"
      n514 = local read "NF_Off_Ref"() -> (w667:refnum<file>)
      n515 = local read "NF_On_Ref"() -> (w668:refnum<file>)
      n516 = local read "FF_Off_Ref"() -> (w669:refnum<file>)
      n517 = local read "FF_On_Ref"() -> (w670:refnum<file>)
      n518 = Close File(refnum=w670) -> ()  [unwired: 1 in, 2 out]
      n519 = Close File(refnum=w669) -> ()  [unwired: 1 in, 2 out]
      n520 = Close File(refnum=w668) -> ()  [unwired: 1 in, 2 out]
      n521 = Close File(refnum=w667) -> ()  [unwired: 1 in, 2 out]
    }
  }
  "FileHour" <- -1 ("FileHour")
  "DataOpen" <- FALSE
